vi "Reliability Project MAIN (PC).vi"() -> ()   [LabVIEW 2019]
uses:
  TypeDef/Test Header.ctl
  TypeDef/Graph Parameters.ctl
  TypeDef/Color.ctl
  TypeDef/Graph Type.ctl
  TypeDef/Graph Output File.ctl
  TypeDef/Test Style.ctl
  TCP/PC/Event Mode.ctl
  TypeDef/Config.ctl
  TypeDef/Test Config.ctl
  TypeDef/Test Parameters.ctl
  <vilib>/Utility/miscctls.llb/LVDateTimeRec.ctl
  TCP/PC/PCsend RTrecv CMD.ctl
  TypeDef/ConnSettingCluster.ctl
  <vilib>/Utility/file.llb/Read Delimited Spreadsheet (DBL).vi
  <vilib>/Utility/config.llb/NI_LVConfig.lvlib
  <vilib>/Utility/config.llb/Write Key (Boolean).vi
  <resource>/objmgr/ni.dex.rc
panel:
  in  "Screen":T1(tab)
  in  "Run Test Tab":enum32{"Page 1"}(tab)
  out "Chart":dbl[][](graph)=[[-0.00241851806640625, 9.5367431640625e-05, 2.3512725830078125, 5.211483001708984, 5.211483001708984], [-0.0020904541015625, 0.0007476806640625, 2.350067138671875, 5.209384918212891, 5.209384918212891], [-0.00305938720703125, 0.00110626220703125, 2.350513458251953, 5.209739685058594, 5.209739685058594], [-0.0022525787353515625, 0.000324249267578125, 2.350391387939453, 5.2073822021484375, 5.2073822021484375], [-0.002140045166015625, 0.0006237030029296875, 2.3496646881103516, 5.206989288330078, 5.206989288330078], [-0.00235748291015625, 0.0009613037109375, 2.349153518676758, 5.206110000610352, 5.206110000610352], [-0.0056972503662109375, -0.000194549560546875, 2.3493595123291016, 5.206518173217773, 5.206518173217773], [-0.002033233642578125, 0.0008106231689453125, 2.347330093383789, 5.203701019287109, 5.203701019287109], [-0.00220489501953125, 0.0001850128173828125, 2.3487815856933594, 5.203361511230469, 5.203361511230469], [-0.002315521240234375, 0.0008544921875, 2.348348617553711, 5.2019500732421875, 5.2019500732421875], [-0.0024318695068359375, 0.0006542205810546875, 2.3473949432373047, 5.201688766479492, 5.201688766479492], [-0.0023937225341796875, 0.0006656646728515625, 2.3465042114257812, 5.199775695800781, 5.199775695800781], [-0.002849578857421875, 0.001049041748046875, 2.346738815307617, 5.199516296386719, 5.199516296386719], [-0.0024662017822265625, 0.001140594482421875, 2.3461246490478516, 5.19781494140625, 5.19781494140625], [-0.0017299652099609375, -0.0011444091796875, 2.3457717895507812, 5.19737434387207, 5.19737434387207], [-0.0023097991943359375, 0.0001659393310546875, 2.345857620239258, 5.196210861206055, 5.196210861206055], [-0.0028095245361328125, 0.0006008148193359375, 2.3449745178222656, 5.195291519165039, 5.195291519165039], [-0.0024776458740234375, 0.0011157989501953125, 2.342325210571289, 5.194158554077148, 5.194158554077148], [-0.0025463104248046875, 0.0005931854248046875, 2.344541549682617, 5.193063735961914, 5.193063735961914], [0.00582122802734375, 8.392333984375e-05, 2.3436336517333984, 5.192634582519531, 5.192634582519531], [-0.004276275634765625, 0.0004634857177734375, 2.3434505462646484, 5.190740585327148, 5.190740585327148], [-0.00257110595703125, 0.0012760162353515625, 2.342508316040039, 5.190359115600586, 5.190359115600586], [-0.0032100677490234375, 0.0006885528564453125, 2.3427352905273438, 5.188653945922852, 5.188653945922852], [-0.0021190643310546875, 0.0008945465087890625, 2.3419570922851562, 5.188499450683594, 5.188499450683594], [-0.0022907257080078125, 0.000335693359375, 2.3421077728271484, 5.186103820800781, 5.186103820800781], [-0.0024394989013671875, 0.0010929107666015625, 2.3413314819335938, 5.186931610107422, 5.186931610107422], [-0.00225830078125, 0.0002803802490234375, 2.3414478302001953, 5.183507919311523, 5.183507919311523], [-0.0024089813232421875, 0.0014781951904296875, 2.340656280517578, 5.184579849243164, 5.184579849243164], [-0.002437591552734375, 0.0005931854248046875, 2.3399314880371094, 5.182092666625977, 5.182092666625977], [-0.002262115478515625, 0.0003643035888671875, 2.3407840728759766, 5.182659149169922, 5.182659149169922], [-0.0025005340576171875, -0.000225067138671875, 2.3396263122558594, 5.1800079345703125, 5.1800079345703125], [-0.00218963623046875, 0.0027942657470703125, 2.338764190673828, 5.180774688720703, 5.180774688720703], [-0.0020732879638671875, 0.0009441375732421875, 2.3374996185302734, 5.177848815917969, 5.177848815917969], [-0.001556396484375, 0.0001373291015625, 2.338285446166992, 5.178548812866211, 5.178548812866211], [-0.0018310546875, 0.0006046295166015625, 2.3379344940185547, 5.175708770751953, 5.175708770751953], [-0.0020771026611328125, 0.0011043548583984375, 2.337373733520508, 5.1764984130859375, 5.1764984130859375], [-0.0024662017822265625, 0.0002307891845703125, 2.3374977111816406, 5.174013137817383, 5.174013137817383], [-0.0022106170654296875, 0.0005321502685546875, 2.336719512939453, 5.174356460571289, 5.174356460571289], [-0.002288818359375, 0.00014495849609375, 2.3338546752929688, 5.171659469604492, 5.171659469604492], [-0.00229644775390625, 0.00081634521484375, 2.335407257080078, 5.172262191772461, 5.172262191772461], [-0.002166748046875, 0.0012416839599609375, 2.327573776245117, 5.169179916381836, 5.169179916381836], [-0.002197265625, 0.000247955322265625, 2.3348464965820312, 5.169887542724609, 5.169887542724609], [-0.002292633056640625, 0.0009975433349609375, 2.334583282470703, 5.167793273925781, 5.167793273925781], [-0.002685546875, 0.0006885528564453125, 2.333953857421875, 5.167308807373047, 5.167308807373047], [-0.002529144287109375, 0.00035858154296875, 2.3336315155029297, 5.165552139282227, 5.165552139282227], [-0.0021762847900390625, 0.0009937286376953125, 2.33294677734375, 5.165216445922852, 5.165216445922852], [-0.002208709716796875, 0.00069427490234375, 2.33135986328125, 5.163597106933594, 5.163597106933594], [-0.0024356842041015625, 0.0005512237548828125, 2.3313236236572266, 5.163679122924805, 5.163679122924805], [-0.002361297607421875, -0.000225067138671875, 2.3319091796875, 5.161943435668945, 5.161943435668945], [-0.0022907257080078125, -0.002529144287109375, 2.3310108184814453, 5.161035537719727, 5.161035537719727], [-0.00202178955078125, 0.0004749298095703125, 2.331541061401367, 5.15962028503418, 5.15962028503418], [-0.00238037109375, -3.0517578125e-05, 2.330432891845703, 5.1588134765625, 5.1588134765625], [-0.001461029052734375, 0.000629425048828125, 2.3308582305908203, 5.157678604125977, 5.157678604125977], [-0.0025424957275390625, 0.0003337860107421875, 2.329559326171875, 5.156576156616211, 5.156576156616211], [-0.002460479736328125, 0.00069427490234375, 2.3291893005371094, 5.156003952026367, 5.156003952026367], [-0.0024356842041015625, 0.001369476318359375, 2.328702926635742, 5.154455184936523, 5.154455184936523], [-0.00209808349609375, 0.00127410888671875, 2.328824996948242, 5.154962539672852, 5.154962539672852], [-0.001079559326171875, 0.0003757476806640625, 2.329326629638672, 5.152063369750977, 5.152063369750977], [-0.0030384063720703125, 0.0001125335693359375, 2.3291149139404297, 5.152074813842773, 5.152074813842773], [-0.0016727447509765625, 5.91278076171875e-05, 2.329296112060547, 5.149860382080078, 5.149860382080078], [-0.002384185791015625, 0.0006103515625, 2.3267383575439453, 5.150243759155273, 5.150243759155273], [-0.00270843505859375, -9.5367431640625e-05, 2.325765609741211, 5.147882461547852, 5.147882461547852], [-0.0021114349365234375, 0.0008640289306640625, 2.325572967529297, 5.148151397705078, 5.148151397705078], [-0.00231170654296875, 0.0012378692626953125, 2.325998306274414, 5.145776748657227, 5.145776748657227], [-0.001338958740234375, 0.0006275177001953125, 2.325258255004883, 5.146303176879883, 5.146303176879883], [-0.0024394989013671875, 0.0006237030029296875, 2.3251724243164062, 5.143526077270508, 5.143526077270508], [-0.0023479461669921875, 0.0012683868408203125, 2.323986053466797, 5.143976211547852, 5.143976211547852], [-0.002422332763671875, 0.0004558563232421875, 2.3242645263671875, 5.1414794921875, 5.1414794921875], [0.0050868988037109375, 0.0001163482666015625, 2.3232860565185547, 5.141656875610352, 5.141656875610352], [-0.0023784637451171875, -2.86102294921875e-05, 2.323179244995117, 5.140108108520508, 5.140108108520508], [-0.0021877288818359375, 0.0002689361572265625, 2.322599411010742, 5.139678955078125, 5.139678955078125], [-0.0022735595703125, 0.000621795654296875, 2.3229293823242188, 5.137945175170898, 5.137945175170898], [-0.002384185791015625, 0.0003204345703125, 2.3215789794921875, 5.137645721435547, 5.137645721435547], [-0.002407073974609375, 0.0003681182861328125, 2.3217506408691406, 5.1365814208984375, 5.1365814208984375], [-0.0019683837890625, 0.000946044921875, 2.3209781646728516, 5.136013031005859, 5.136013031005859], [-0.002208709716796875, 0.000820159912109375, 2.320514678955078, 5.134279251098633, 5.134279251098633], [-0.002262115478515625, 0.0007038116455078125, 2.320322036743164, 5.133800506591797, 5.133800506591797], [-0.0022068023681640625, 0.000804901123046875, 2.3203296661376953, 5.132570266723633, 5.132570266723633], [-0.0026531219482421875, 0.000782012939453125, 2.318910598754883, 5.131275177001953, 5.131275177001953], [-0.0024929046630859375, 0.00089263916015625, 2.3195762634277344, 5.130367279052734, 5.130367279052734], [-0.00217437744140625, 0.000827789306640625, 2.3187484741210938, 5.129323959350586, 5.129323959350586], [-0.0023651123046875, 0.0007495880126953125, 2.3187007904052734, 5.128835678100586, 5.128835678100586], [-0.0020999908447265625, 0.00095367431640625, 2.3181400299072266, 5.127468109130859, 5.127468109130859], [-0.0024890899658203125, 0.0009746551513671875, 2.3181591033935547, 5.12727165222168, 5.12727165222168], [-0.0021305084228515625, 0.00098419189453125, 2.3174896240234375, 5.125310897827148, 5.125310897827148], [-0.002712249755859375, 0.0005664825439453125, 2.3167991638183594, 5.125190734863281, 5.125190734863281], [-0.0021343231201171875, 0.0006313323974609375, 2.3164443969726562, 5.123414993286133, 5.123414993286133], [-0.0029354095458984375, 0.0004596710205078125, 2.3162708282470703, 5.123697280883789, 5.123697280883789], [-0.00228118896484375, -7.62939453125e-06, 2.3158607482910156, 5.121555328369141, 5.121555328369141], [-0.0022182464599609375, 0.0007076263427734375, 2.3154754638671875, 5.12164306640625, 5.12164306640625], [-0.002349853515625, 0.0007724761962890625, 2.315549850463867, 5.119346618652344, 5.119346618652344], [-0.002269744873046875, 0.001094818115234375, 2.3123722076416016, 5.119991302490234, 5.119991302490234], [-0.00231170654296875, 0.0002613067626953125, 2.3144569396972656, 5.117624282836914, 5.117624282836914], [-0.00157928466796875, 0.000156402587890625, 2.313823699951172, 5.118106842041016, 5.118106842041016], [-0.0027179718017578125, 0.0005702972412109375, 2.314136505126953, 5.115741729736328, 5.115741729736328], [-0.0025234222412109375, 3.814697265625e-06, 2.312936782836914, 5.116338729858398, 5.116338729858398], [-0.002349853515625, 0.0016937255859375, 2.3126564025878906, 5.113800048828125, 5.113800048828125], [-0.0027751922607421875, 0.0006504058837890625, 2.312501907348633, 5.1144256591796875, 5.1144256591796875], [-0.002429962158203125, 0.00086212158203125, 2.31304931640625, 5.112766265869141, 5.112766265869141], [-0.0024261474609375, 0.0006504058837890625, 2.3119125366210938, 5.112785339355469, 5.112785339355469], [-0.0024738311767578125, -1.33514404296875e-05, 2.3113555908203125, 5.110126495361328, 5.110126495361328], [-0.002063751220703125, 4.76837158203125e-05, 2.308307647705078, 5.110754013061523, 5.110754013061523], [-0.00232696533203125, -6.103515625e-05, 2.31024169921875, 5.108325958251953, 5.108325958251953], [-0.002197265625, 0.00018310546875, 2.3096885681152344, 5.109380722045898, 5.109380722045898], [-0.0021686553955078125, 0.000545501708984375, 2.3098373413085938, 5.106624603271484, 5.106624603271484], [-0.0011692047119140625, 0.000392913818359375, 2.309000015258789, 5.107295989990234, 5.107295989990234], [-0.0025653839111328125, 0.0001506805419921875, 2.3094406127929688, 5.105155944824219, 5.105155944824219], [-0.002166748046875, 0.000545501708984375, 2.3088741302490234, 5.105400085449219, 5.105400085449219], [-0.00229644775390625, 0.000518798828125, 2.3076095581054688, 5.102983474731445, 5.102983474731445], [-0.0026874542236328125, 0.00115966796875, 2.3078269958496094, 5.103851318359375, 5.103851318359375], [-0.0022907257080078125, 0.0001049041748046875, 2.308218002319336, 5.101722717285156, 5.101722717285156], [-0.0018825531005859375, 0.000579833984375, 2.3090286254882812, 5.102010726928711, 5.102010726928711], [-0.002620697021484375, 0.000263214111328125, 2.3078346252441406, 5.100181579589844, 5.100181579589844], [-0.0020904541015625, 0.000461578369140625, 2.3070220947265625, 5.09980583190918, 5.09980583190918], [-0.002315521240234375, 8.96453857421875e-05, 2.2959556579589844, 5.099071502685547, 5.099071502685547], [-0.0024433135986328125, -3.4332275390625e-05, 2.306089401245117, 5.098339080810547, 5.098339080810547], [-0.0015163421630859375, 1.52587890625e-05, 2.305643081665039, 5.097761154174805, 5.097761154174805], [-0.00197601318359375, 0.0005550384521484375, 2.305318832397461, 5.096200942993164, 5.096200942993164], [-0.002300262451171875, 0.0008144378662109375, 2.3057098388671875, 5.096399307250977, 5.096399307250977], [-0.0022907257080078125, 0.001064300537109375, 2.304637908935547, 5.094629287719727, 5.094629287719727], [-0.0023441314697265625, 0.000896453857421875, 2.3045883178710938, 5.094669342041016, 5.094669342041016], [-0.0025272369384765625, 0.0006122589111328125, 2.3042259216308594, 5.092912673950195, 5.092912673950195], [-0.002017974853515625, 0.000339508056640625, 2.303884506225586, 5.093050003051758, 5.093050003051758], [-0.0024871826171875, 0.000335693359375, 2.3036632537841797, 5.091398239135742, 5.091398239135742], [-0.0026378631591796875, 0.0004863739013671875, 2.291349411010742, 5.092126846313477, 5.092126846313477], [-0.0020580291748046875, 0.0008220672607421875, 2.303516387939453, 5.089519500732422, 5.089519500732422], [-0.0019683837890625, 0.0003223419189453125, 2.302806854248047, 5.090400695800781, 5.090400695800781], [-0.00337982177734375, 0.0012302398681640625, 2.3025283813476562, 5.087850570678711, 5.087850570678711], [-0.0022869110107421875, 0.0002040863037109375, 2.299816131591797, 5.088750839233398, 5.088750839233398], [-0.0024471282958984375, 0.0006580352783203125, 2.302255630493164, 5.086374282836914, 5.086374282836914], [-0.0022602081298828125, 0.0002288818359375, 2.301565170288086, 5.087335586547852, 5.087335586547852], [-0.002094268798828125, -3.4332275390625e-05, 2.300901412963867, 5.085031509399414, 5.085031509399414], [-0.0021820068359375, 0.0004425048828125, 2.300508499145508, 5.085823059082031, 5.085823059082031], [-0.003513336181640625, -0.00026702880859375, 2.3003177642822266, 5.0836639404296875, 5.0836639404296875], [-0.0021228790283203125, 0.00023651123046875, 2.299711227416992, 5.084384918212891, 5.084384918212891], [-0.0023136138916015625, 7.62939453125e-05, 2.3003311157226562, 5.082035064697266, 5.082035064697266], [-0.002285003662109375, 2.288818359375e-05, 2.2995033264160156, 5.083127975463867, 5.083127975463867], [-0.0023632049560546875, 0.00054931640625, 2.2997283935546875, 5.080684661865234, 5.080684661865234], [-0.0022487640380859375, 0.000881195068359375, 2.299091339111328, 5.081302642822266, 5.081302642822266], [-0.00244903564453125, 0.0009021759033203125, 2.2994842529296875, 5.079761505126953, 5.079761505126953], [-0.00209808349609375, 0.000762939453125, 2.2970943450927734, 5.080654144287109, 5.080654144287109], [-0.0023212432861328125, 4.38690185546875e-05, 2.3003578186035156, 5.078205108642578, 5.078205108642578], [-0.0018157958984375, 0.0008544921875, 2.2980213165283203, 5.078620910644531, 5.078620910644531], [-0.0022640228271484375, 0.0011501312255859375, 2.2982006072998047, 5.0772857666015625, 5.0772857666015625], [-0.0029888153076171875, 0.0002002716064453125, 2.298887252807617, 5.07684326171875, 5.07684326171875], [-0.0024242401123046875, 0.0006103515625, 2.2978076934814453, 5.075416564941406, 5.075416564941406], [-0.0022754669189453125, 0.0011653900146484375, 2.297220230102539, 5.0757904052734375, 5.0757904052734375], [-0.001163482666015625, 0.0010986328125, 2.297616958618164, 5.07489013671875, 5.07489013671875], [-0.002658843994140625, 0.0008525848388671875, 2.2969589233398438, 5.074573516845703, 5.074573516845703], [-0.0022487640380859375, 0.0010128021240234375, 2.2956104278564453, 5.073554992675781, 5.073554992675781], [-0.0024967193603515625, 0.0009746551513671875, 2.296297073364258, 5.073375701904297, 5.073375701904297], [-0.0025348663330078125, -0.0001773834228515625, 2.2911739349365234, 5.07227897644043, 5.07227897644043], [-0.0026683807373046875, 0.00122833251953125, 2.297945022583008, 5.072353363037109, 5.072353363037109], [-0.0019474029541015625, 0.0010662078857421875, 2.2958545684814453, 5.071252822875977, 5.071252822875977], [-0.002422332763671875, 0.000732421875, 2.295177459716797, 5.071023941040039, 5.071023941040039], [-0.00240325927734375, -0.0006256103515625, 2.295278549194336, 5.070167541503906, 5.070167541503906], [-0.00270843505859375, 0.0004940032958984375, 2.2949085235595703, 5.070009231567383, 5.070009231567383], [-0.0024509429931640625, 0.0009822845458984375, 2.295053482055664, 5.06922721862793, 5.06922721862793], [-0.0033931732177734375, 3.4332275390625e-05, 2.294820785522461, 5.068716049194336, 5.068716049194336], [-0.0019702911376953125, 0.0010128021240234375, 2.2952404022216797, 5.068096160888672, 5.068096160888672], [-0.0023193359375, 0.0004405975341796875, 2.294109344482422, 5.067258834838867, 5.067258834838867], [-0.0024013519287109375, 0.00025177001953125, 2.2938690185546875, 5.067533493041992, 5.067533493041992], [-0.00215911865234375, 0.00032806396484375, 2.2927303314208984, 5.066440582275391, 5.066440582275391], [-0.001934051513671875, 0.000698089599609375, 2.2940006256103516, 5.066160202026367, 5.066160202026367], [-0.00247955322265625, 0.0002422332763671875, 2.293081283569336, 5.065158843994141, 5.065158843994141], [-0.00244903564453125, 0.0005702972412109375, 2.292530059814453, 5.065837860107422, 5.065837860107422], [-0.002269744873046875, 0.00032806396484375, 2.2919998168945312, 5.064092636108398, 5.064092636108398], [-0.0024890899658203125, 0.0002803802490234375, 2.292816162109375, 5.064476013183594, 5.064476013183594], [-0.0021076202392578125, 0.0007839202880859375, 2.2923927307128906, 5.063138961791992, 5.063138961791992], [-0.0026073455810546875, 0.0004119873046875, 2.292522430419922, 5.0640716552734375, 5.0640716552734375], [-0.0022125244140625, 0.0003604888916015625, 2.292064666748047, 5.061803817749023, 5.061803817749023], [-0.0021190643310546875, 0.00043487548828125, 2.291830062866211, 5.063020706176758, 5.063020706176758], [-0.0026988983154296875, -8.58306884765625e-05, 2.291942596435547, 5.060863494873047, 5.060863494873047], [-0.0024967193603515625, 0.0013103485107421875, 2.2912254333496094, 5.062192916870117, 5.062192916870117], [-0.0023708343505859375, 0.0013580322265625, 2.290983200073242, 5.060268402099609, 5.060268402099609], [-0.0019283294677734375, 0.0005130767822265625, 2.2912445068359375, 5.0613250732421875, 5.0613250732421875], [-0.00235748291015625, 0.0006389617919921875, 2.291158676147461, 5.059490203857422, 5.059490203857422], [-0.0021953582763671875, 0.0008640289306640625, 2.290618896484375, 5.060487747192383, 5.060487747192383], [-0.002262115478515625, 0.0003376007080078125, 2.2910594940185547, 5.058900833129883, 5.058900833129883], [-0.004283905029296875, 0.0003986358642578125, 2.2887744903564453, 5.059345245361328, 5.059345245361328], [-0.0024280548095703125, 0.00084686279296875, 2.2905349731445312, 5.057645797729492, 5.057645797729492], [-0.0024051666259765625, 0.001026153564453125, 2.289949417114258, 5.0586395263671875, 5.0586395263671875], [-0.00244140625, 0.0017452239990234375, 2.2903308868408203, 5.056642532348633, 5.056642532348633], [-0.0020580291748046875, 0.0011138916015625, 2.2884883880615234, 5.057493209838867, 5.057493209838867], [-0.00202178955078125, 0.0007648468017578125, 2.2892799377441406, 5.055974960327148, 5.055974960327148], [-0.0024394989013671875, -8.7738037109375e-05, 2.289255142211914, 5.057348251342773, 5.057348251342773], [-0.0016193389892578125, 0.0003337860107421875, 2.288480758666992, 5.055501937866211, 5.055501937866211], [-0.0021190643310546875, 0.000507354736328125, 2.2884178161621094, 5.056310653686523, 5.056310653686523], [-0.002429962158203125, 0.001087188720703125, 2.2895164489746094, 5.05482292175293, 5.05482292175293], [-0.002117156982421875, 0.000701904296875, 2.2885704040527344, 5.055061340332031, 5.055061340332031], [-0.0021724700927734375, 0.000560760498046875, 2.2890186309814453, 5.054107666015625, 5.054107666015625], [-0.002399444580078125, 0.00107574462890625, 2.2880687713623047, 5.054941177368164, 5.054941177368164], [-0.00286865234375, 0.000347137451171875, 2.288494110107422, 5.053903579711914, 5.053903579711914], [-0.0020732879638671875, 0.000972747802734375, 2.288127899169922, 5.053012847900391, 5.053012847900391], [-0.00222015380859375, 0.0010051727294921875, 2.2885360717773438, 5.053804397583008, 5.053804397583008], [-0.002368927001953125, 0.0002231597900390625, 2.288074493408203, 5.053201675415039, 5.053201675415039], [-0.0024871826171875, 0.0008525848388671875, 2.28802490234375, 5.0528564453125, 5.0528564453125], [-0.00225067138671875, 0.0009307861328125, 2.2883853912353516, 5.052770614624023, 5.052770614624023], [-0.0021457672119140625, 0.0007495880126953125, 2.287994384765625, 5.051923751831055, 5.051923751831055], [-0.0021305084228515625, 0.0013179779052734375, 2.28741455078125, 5.051168441772461, 5.051168441772461]]
  in  "pb.graph control":bool caption="Digital Output 4"
  in  "pb.RunSweeps":bool caption="Start Sweeps"
  out "Abs. Height":dbl
  out "PS Volt":dbl
  out "LS Volt":dbl
  out "Spare":dbl
  in  "Sweep Time (s)":dbl min=0.0 step=0.01 format="%.2g"
  in  "Sweep End Height":dbl
  in  "Number of Sweeps":i32
  out "Data Path":path
  in  "Sweep Start Height":dbl
  in  "Sweep PS Cmd":dbl
  out "Resistance":dbl=nan
  out "Sweeps Complete":i16
  out "Min Height":dbl
  out "Max Height":dbl
  in  "Spare Output":dbl
  in  "PS Command":dbl
  in  "Position Command":dbl=nan
  in  "pb.TareHeight":bool caption="Start Sweeps"
  out "Relative Height":dbl format="%#.3g"
  in  "Test Setup Tab":enum32{"Page 1"}(tab)
  in  "pb.Open Test Config":bool caption="Copy Test Setup"
  out "Test Config":string
  in  "Test Style":T2
  in  "Bias Resistance":dbl=nan
  in  "pb.Copy Test Config":bool caption="Copy Test Setup"
  in  "Graph Setup Tab":enum32{"Page 1"}(tab)
  in  "pb.Graph by File":bool caption="Digital Output 4"
  in  "pb.Re-Run Graph":bool caption="Digital Output 4"
  in  "Graph Parameters":T3={"Tol Path"=path "", "Tol Band Color"=enum."Red", "Graph Type"=enum."H vs R (1 Cycle)", "Height Min"=0, "Height Max"=0, "Height Interval"=0, "Res Max"=0, "Res Interval"=0, "Time Max"=0, "Time Interval"=0, "Graph Output File"=enum."pdf", "Auto Open"=TRUE}
  in  "Test Header Tab":enum32{"Page 1"}(tab)
  in  "Test Header":T7
  out "led.DataWarning":bool=TRUE caption="Check last file for missing data\n          (jumps in height)"
  in  "pb.CalPage":bool caption="Digital Output 4"
  out "IP Address":string
  in  "pb.connect":bool
  out "InvalidResponses":string
  out "Error Out":errorcluster
  in  "FlattenedData":string
  in  "Command":string
  in  "Connected?":bool
  in  "Connected? 2":bool
  in  "Panel Close?":bool
  in  "pb.DO0":bool caption="Digital Output 1"
  in  "pb.DO1":bool caption="Digital Output 2"
  in  "pb.DO2":bool caption="Digital Output 3"
  in  "pb.DO3":bool caption="Digital Output 4"
  out "led.DI 4":bool caption="Digital Input 1"
  out "led.DI 5":bool caption="Digital Input 2"
  out "led.DI 6":bool caption="Digital Input 3"
  out "led.DI 7":bool caption="Digital Input 4"
  in  "Cal Due Date:":timestamp=timestamp(3029616000 s since 1904-01-01) format="%<%m/%d/%y>T"
  in  "Gauge Number:":i32[](array[numeric])=[0, 0, 0, 0, 0, 0, 0]
  out "Cal Readings:":dbl[](array[numeric])
  in  "Cal Controls:":dbl[](array[numeric])=[nan, 0.0, 0.0]
  in  "pb.RevertCal":bool
  in  "pb.SaveCal":bool
  out "Channels:":string[](array[string])=["Power Supply Voltage", "Level Sender Voltage", "AI-3 Spare", "Height Gauge", "Position Command", "Power Supply Command", "Spare Output"]
  in  "Offset Values:":dbl[](array[numeric])=[0.0, 0.0, 0.0, 0.0, 0.0, 0.0, 0.0]
  in  "Slope Values:":dbl[](array[numeric])=[0.0, 0.0, 0.0, 0.0, 0.0, 0.0, 0.0]
  in  "pb.RunScreen":bool caption="Digital Output 4"
  # "Run Test"
  # "Test Setup"
  # "Graph Setup"
  # "Test Header"
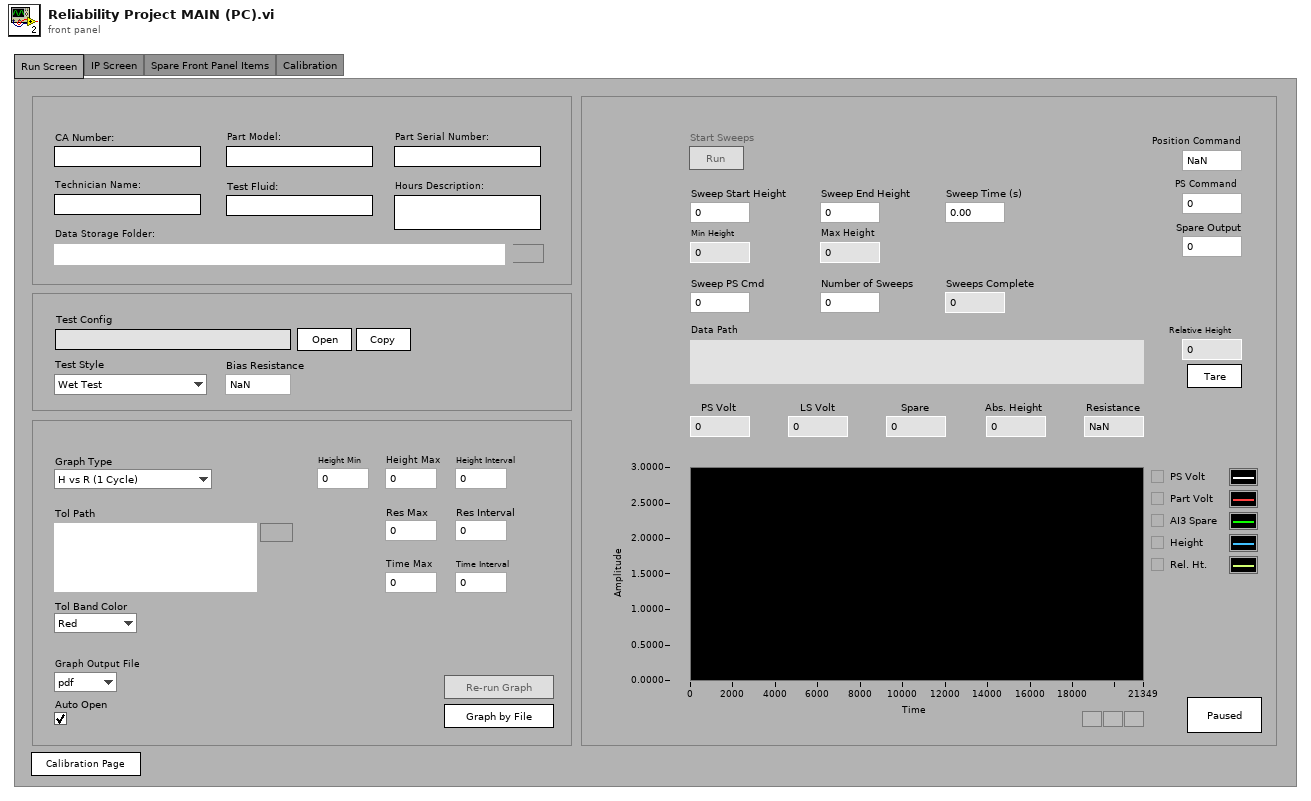
[diagram p1: front panel]
types:
  T1 = enum32{"Run Screen", "IP Screen", "Spare Front Panel Items", "Calibration"}
  T2 = typedef "Test Style.ctl" = enum16{"Wet Test", "Dry Test", "Contact Test"}
  T3 = typedef "Graph Parameters.ctl" = cluster{"Tol Path":path, "Tol Band Color":T4, "Graph Type":T5, "Height Min":i32, "Height Max":i32, "Height Interval":i32, "Res Max":i32, "Res Interval":i32, "Time Max":i32, "Time Interval":i32, "Graph Output File":T6, "Auto Open":bool}
  T4 = typedef "Color.ctl" = enum16{"Red", "Black", "Green", "Blue", "Orange", "Yellow", "Purple", "Grey"}
  T5 = typedef "Graph Type.ctl" = enum16{"H vs R (1 Cycle)", "T vs R (Multiple Cycles)", "H vs R & T vs R (1 Cycle)"}
  T6 = typedef "Graph Output File.ctl" = enum16{"png", "pdf"}
  T7 = typedef "Test Header.ctl" = cluster{"CA Number:":string, "Part Model:":string, "Part Serial Number:":string, "Technician Name:":string, "Test Fluid:":string, "Hours Description:":string, "Data Storage Folder:":path}
  T8 = typedef "Test Config.ctl" = cluster{"Test Header":T7, "Test Style":T2, "Bias Resistance":dbl, "Height Offset":dbl, "Graph Parameters":T3, "Test Parameters":T9}
  T9 = typedef "Test Parameters.ctl" = cluster{"Sweep Start Height":dbl, "Sweep End Height":dbl, "Sweep Time (s)":dbl, "Sweep PS Cmd":dbl, "Number of Sweeps":i32}
  T10 = typedef "Config.ctl" = cluster{"Test Config Path":path, "RT IP Address":string}
  T11 = typedef "Event Mode.ctl" = enum16{"Init", "Get", "Set", "Destroy"}
  T12 = cluster{"Config":T10, "RIOTries":i32, "RIOconnection":bool, "IP Address":string, "ValidFile?":bool, "Graph Active":bool, "Data Clock":dbl, "Data Timing":dbl, "Data":dbl[][], "Data_Current":dbl[], "Slope Values":dbl[], "Offset Values":dbl[], "Controls":dbl[], "Height Offset":dbl, "Data Path":path, "SweepsRunning":bool, "SweepsForward":bool, "SweepsSwept":i32, "Gauge#":i32, "CalDueDate":string, "Data Index":i32, "Sweep Clock":dbl, "Sweep Timing":dbl, "Waveform":dbl[], "Wave.pts":i32, "Current Point":i32, "FinalizeSweeps":bool, "New Data":bool, "MaxResistance":dbl, "Min Height":dbl, "Max Height":dbl, "Graph Time":dbl, "Config Path":path, "Time v Res":bool, "Test Params":T8, "Test Config":string, "Graphing Script Dir":path, "Graph Data":dbl[][]}
  T13 = typedef "LVDateTimeRec.ctl" = cluster{"fractional second":dbl, "second":i32, "minute":i32, "hour":i32, "day of month":i32, "month":i32, "year":i32, "day of week":i32, "day of year":i32, "DST":i32}
  T14 = typedef "PCsend RTrecv CMD.ctl" = enum16{"ConnSettings", "Connect", "Stop", "Digital Outputs", "Analog Outputs", "Sweep Parameters", "Start Sweep", "Cal2RT", "Save Cal", "Load Cal"}
  T15 = enum32{"Run Screen", "IP Screen", "Spare Front Panel Items", "Calibration", "New LS"}
  T16 = enum32{"invalid app kind", "Development System", "Run Time System", "Student Edition", "Embedded LabVIEW", "Evaluation", "Custom"}
  T17 = enum16{"Read Data", "Write Data", "Write Cal", "Init", "Write Stream Error"}
  T18 = cluster{"Slope":dbl[], "Offset":dbl[], "Gauge#":i32, "CalDueDate":string}
  T19 = enum16{"open", "replace", "create", "open or create", "replace or create", "replace or create with confirmation"}
  T20 = enum8{"Enabled", "Disabled", "Disabled and Grayed Out"}
  T21 = enum32{"Run Screen", "Test Configuration Page", "Stand Configuration Page", "RIO Connection", "Part Change", "Spare Front Panel Items", "Intro", "Cal Warning"}
  T22 = typedef "RTsend PCrecv CMD.ctl" = enum16{"Digital Inputs", "Connected?", "Data", "Data 2", "Cal2PC"}
  T23 = cluster{"Slope Values":dbl[], "Offset Values":dbl[]}
  T24 = cluster{"Numeric":i32, "date/time string":string}
  T25 = typedef "NI_LVConfig.lvlib/Config Data RefNum.ctl" = refnum<k1>
  T26 = typedef "ConnSettingCluster.ctl" = cluster{"ConnectAttemptLimit(5)":u32, "IP Address":string, "Send Port":u16, "Recv Port":u16}
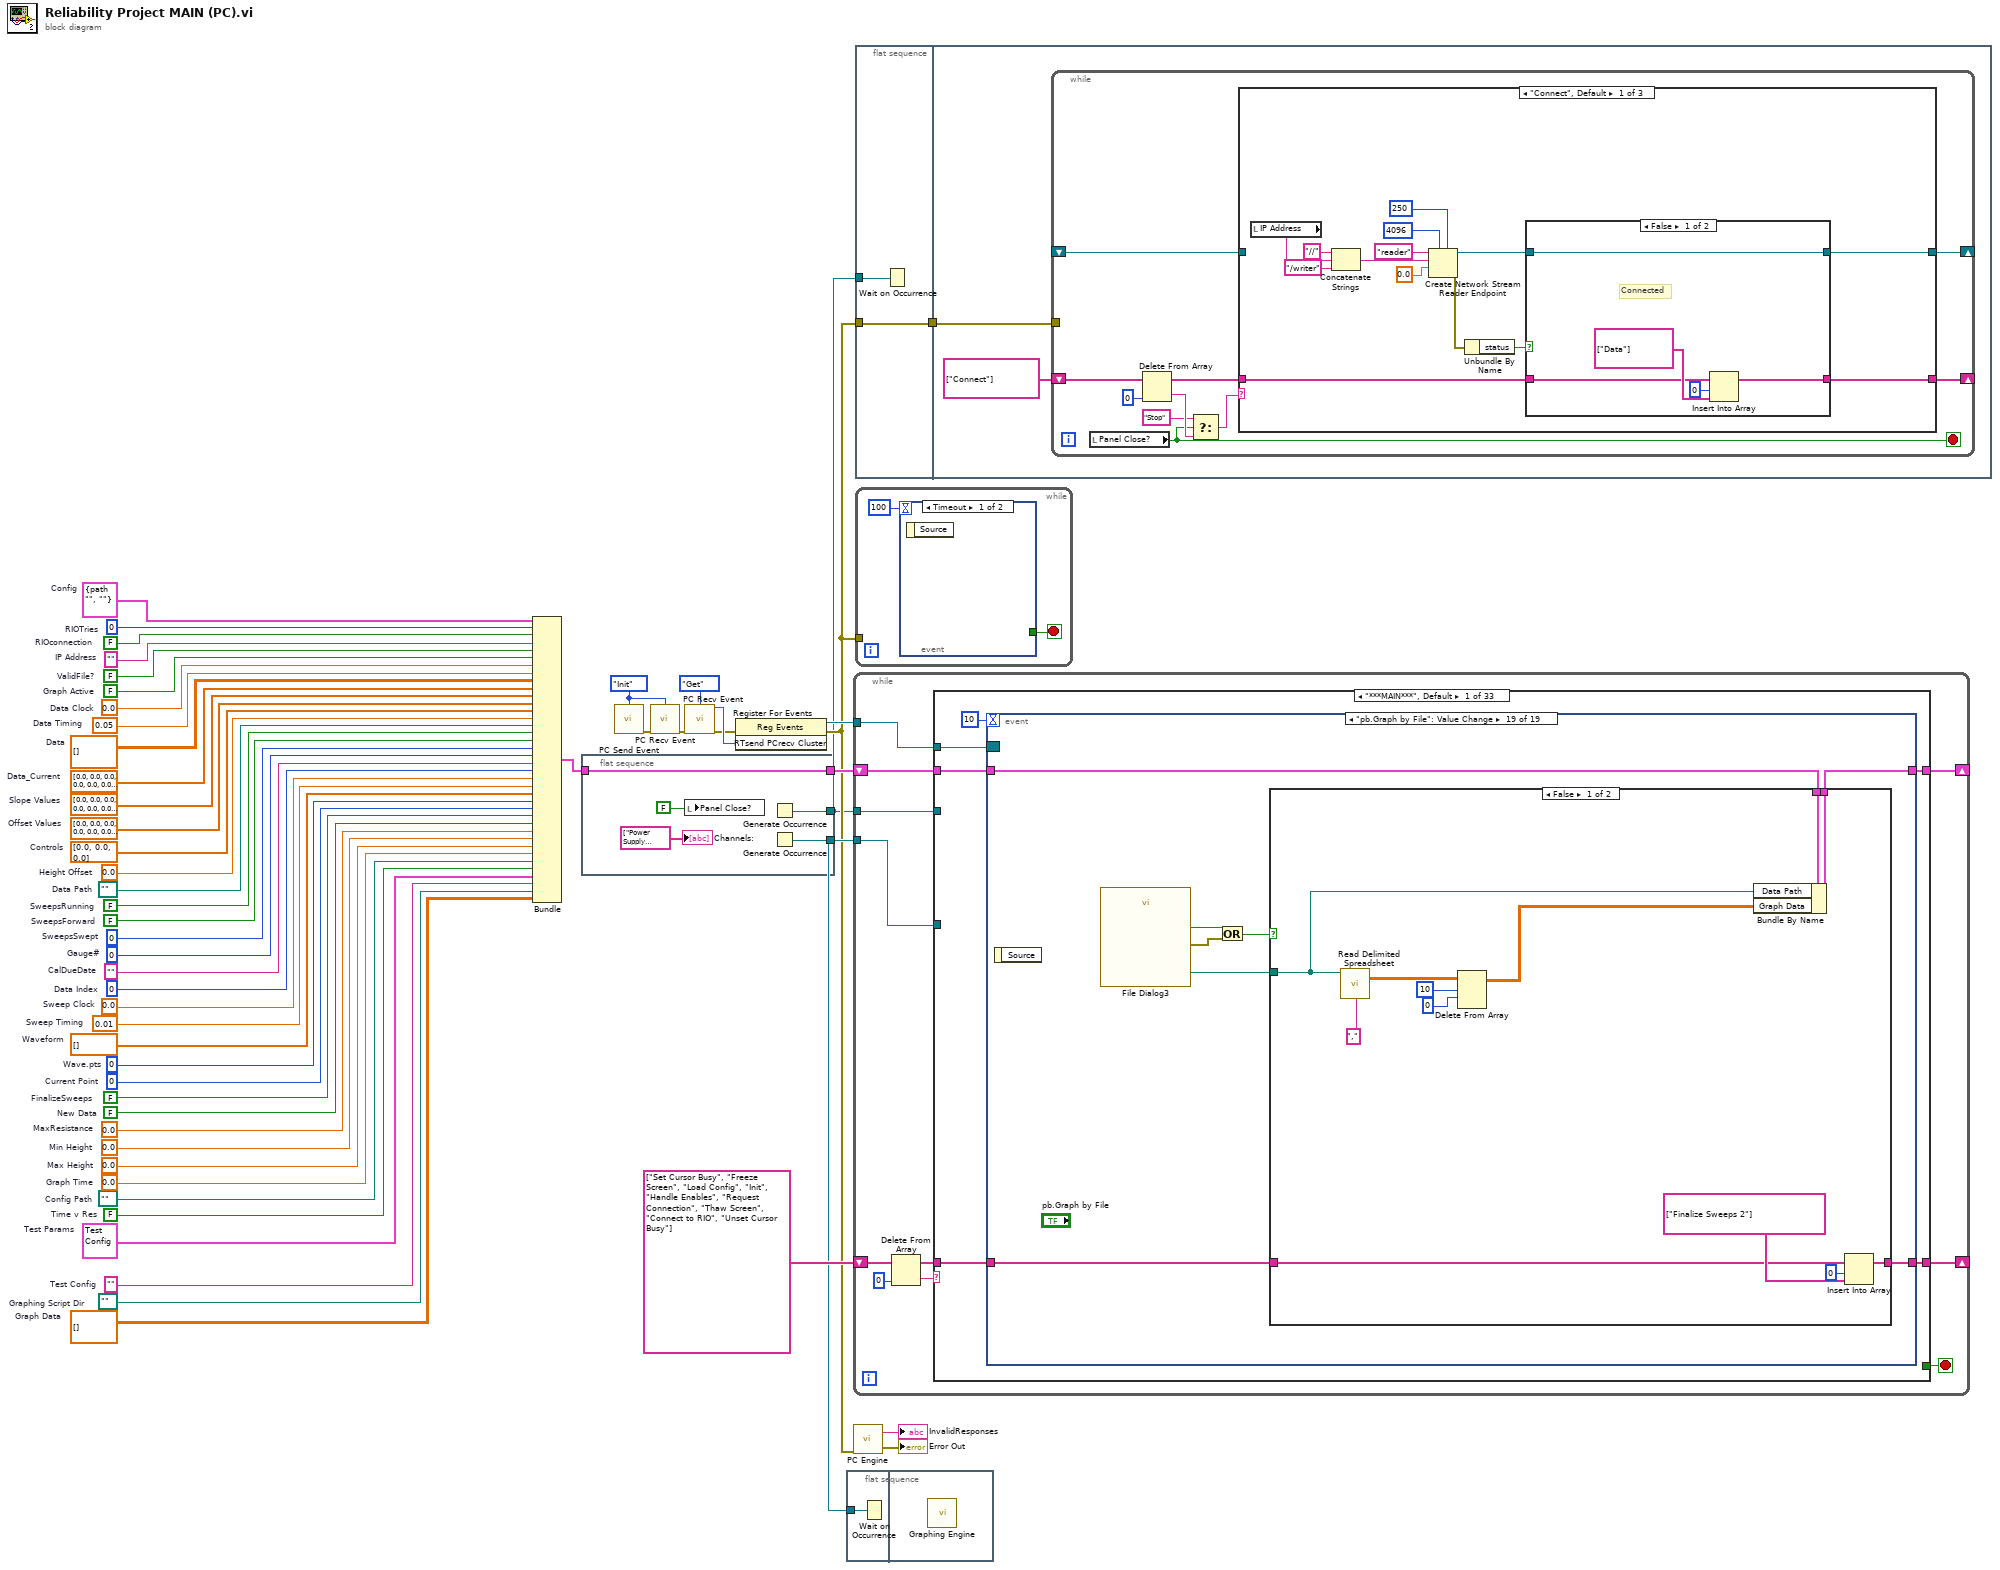
[diagram p0: block diagram]
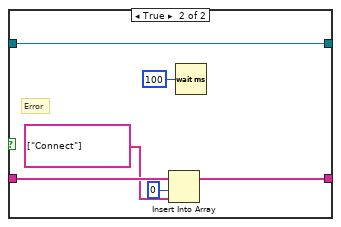
[diagram p2: hidden frame]
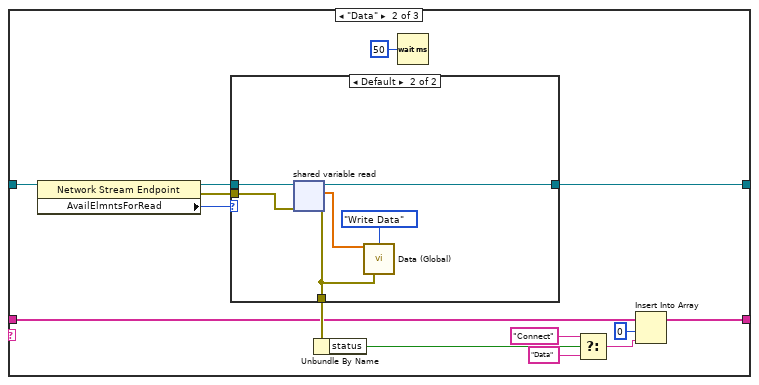
[diagram p3: hidden frame]
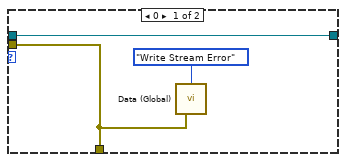
[diagram p4: hidden frame]
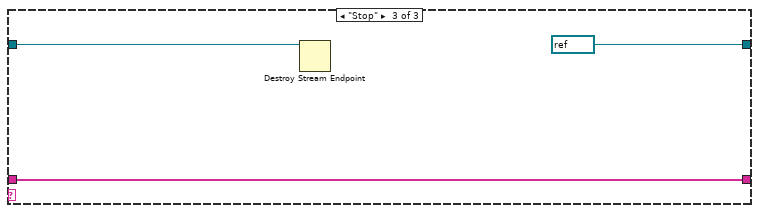
[diagram p5: hidden frame]
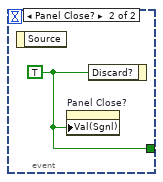
[diagram p6: hidden frame]
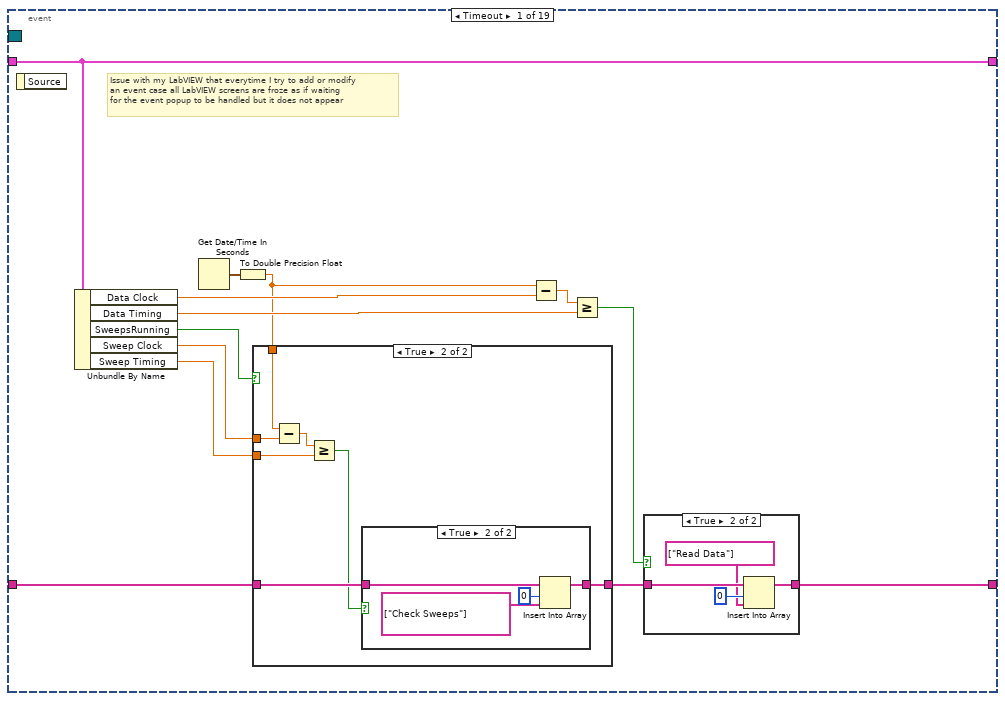
[diagram p7: hidden frame]
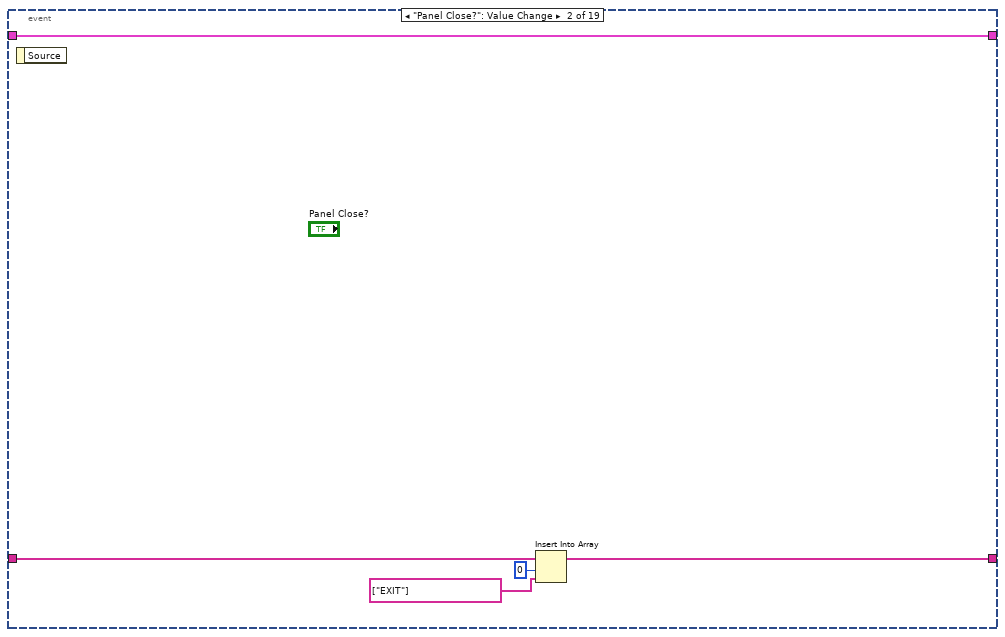
[diagram p11: hidden frame]
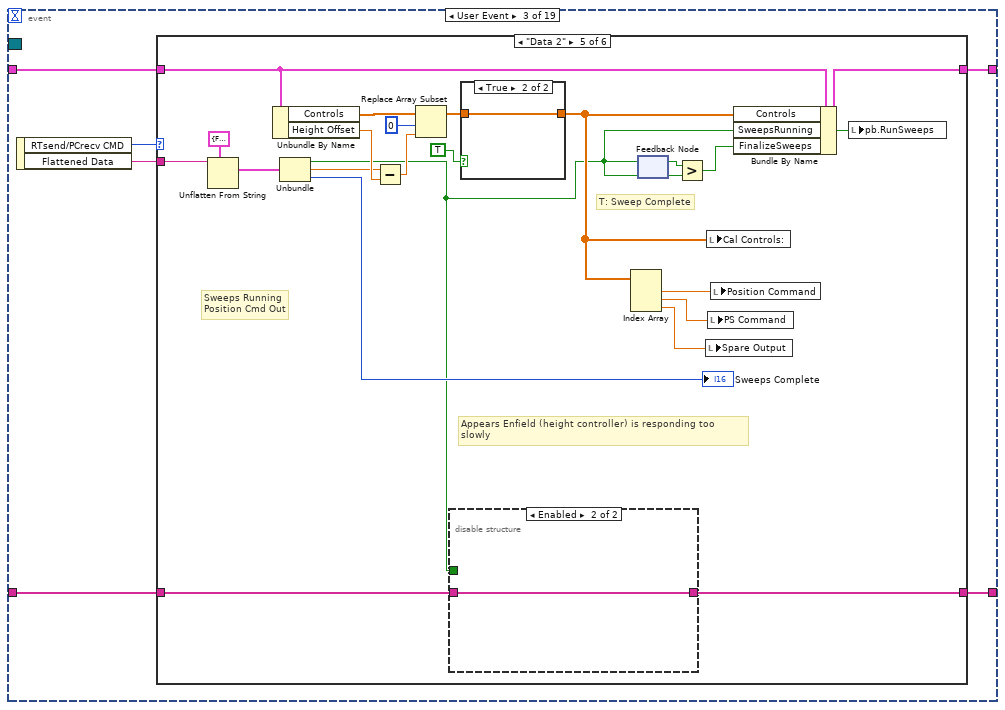
[diagram p12: hidden frame]
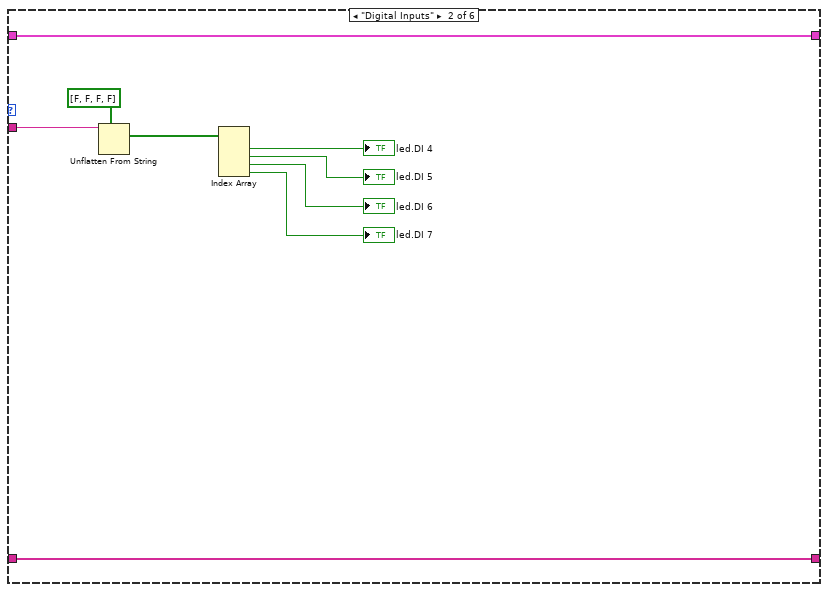
[diagram p14: hidden frame]
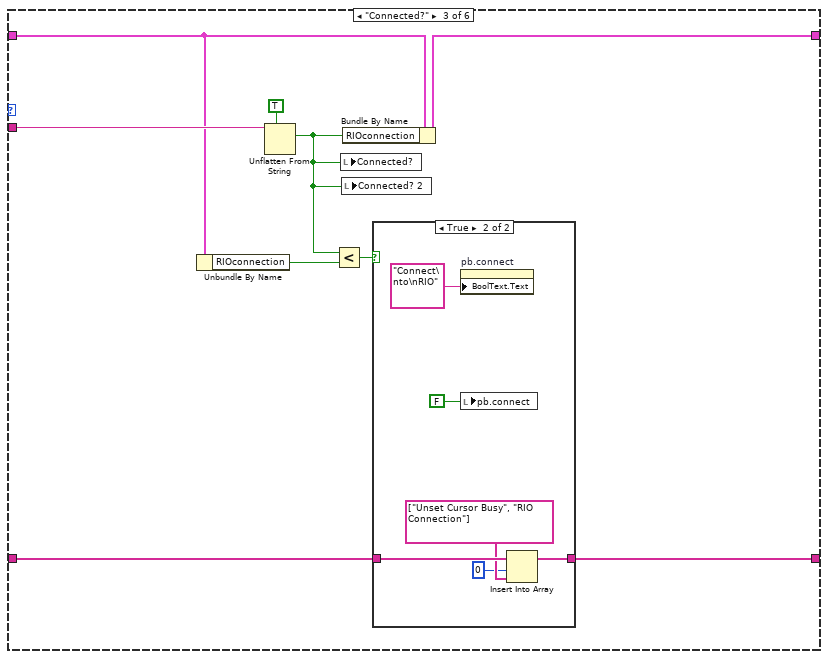
[diagram p15: hidden frame]
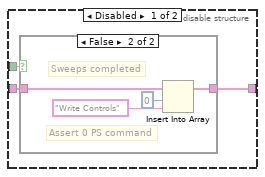
[diagram p18: hidden frame]
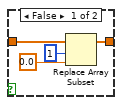
[diagram p20: hidden frame]
diagram:
  w1 = dbl[][] []  # Graph Data
  w2 = path ""  # Graphing Script Dir
  w3 = ""  # Test Config
  w4 = T8 {"Test Header"={"CA Number:"="", "Part Model:"="", "Part Serial Number:"="", "Technician Name:"="", "Test Fluid:"="", "Hours Description:"="", "Data Storage Folder:"=path ""}, "Test Style"=enum."Wet Test", "Bias Resistance"=nan, "Height Offset"=nan, "Graph Parameters"={"Tol Path"=path "C:/Users/gtetil/Documents/Projects/Reliability-Sweeper/Source/Files/Graphing Script/E7x Tolerance (MS, dry).csv", "Tol Band Color"=enum."Red", "Graph Type"=enum."H vs R & T vs R (1 Cycle)", "Height Min"=-15, "Height Max"=250, "Height Interval"=50, "Res Max"=1250, "Res Interval"=100, "Time Max"=10, "Time Interval"=1, "Graph Output File"=enum."pdf", "Auto Open"=TRUE}, "Test Parameters"={"Sweep Start Height"=0.0, "Sweep End Height"=0.0, "Sweep Time (s)"=0.0, "Sweep PS Cmd"=0.0, "Number of Sweeps"=0}}  # Test Params
  w5 = FALSE  # Time v Res
  w6 = path ""  # Config Path
  w7 = T10 {"Test Config Path"=path "", "RT IP Address"=""}  # Config
  w8 = 0.0  # Graph Time
  w13 = 0.0  # Max Height
  w14 = 0.0  # Min Height
  w15 = 0.0  # MaxResistance
  w16 = FALSE  # New Data
  w17 = FALSE  # FinalizeSweeps
  w20 = 0  # Current Point
  w19 = 0  # Wave.pts
  w18 = dbl[] []  # Waveform
  w21 = 0.01  # Sweep Timing
  w22 = 0.0  # Sweep Clock
  w23 = 0  # Data Index
  w25 = 0  # Gauge#
  w24 = ""  # CalDueDate
  w26 = dbl[] [0.0, 0.0, 0.0, 0.0, 0.0, 0.0, 0.0]  # Data_Current
  w28 = 0  # SweepsSwept
  w29 = FALSE  # SweepsForward
  w30 = FALSE  # SweepsRunning
  w31 = path ""  # Data Path
  w32 = 0.0  # Height Offset
  w33 = dbl[] [0.0, 0.0, 0.0]  # Controls
  w27 = dbl[] [0.0, 0.0, 0.0, 0.0, 0.0, 0.0, 0.0]  # Slope Values
  w34 = dbl[] [0.0, 0.0, 0.0, 0.0, 0.0, 0.0, 0.0]  # Offset Values
  w35 = dbl[][] []  # Data
  w36 = 0.05  # Data Timing
  w37 = 0.0  # Data Clock
  w38 = FALSE  # Graph Active
  w45 = Event_Mode."Init" ("Mode")
  w51 = FALSE  # ValidFile?
  w52 = ""  # IP Address
  w53 = 0  # RIOTries
  w54 = FALSE  # RIOconnection
  n1 = Bundle("Config"=w7, "RIOTries"=w53, "RIOconnection"=w54, "IP Address"=w52, "ValidFile?"=w51, "Graph Active"=w38, "Data Clock"=w37, "Data Timing"=w36, "Data"=w35, "Data_Current"=w26, "Slope Values"=w27, "Offset Values"=w34, "Controls"=w33, "Height Offset"=w32, "Data Path"=w31, "SweepsRunning"=w30, "SweepsForward"=w29, "SweepsSwept"=w28, "Gauge#"=w25, "CalDueDate"=w24, "Data Index"=w23, "Sweep Clock"=w22, "Sweep Timing"=w21, "Waveform"=w18, "Wave.pts"=w19, "Current Point"=w20, "FinalizeSweeps"=w17, "New Data"=w16, "MaxResistance"=w15, "Min Height"=w14, "Max Height"=w13, "Graph Time"=w8, "Config Path"=w6, "Time v Res"=w5, "Test Params"=w4, "Test Config"=w3, "Graphing Script Dir"=w2, "Graph Data"=w1) -> (w50:T12)  [unwired: 1 in]
  n2 = flat-sequence {
    tunnel: w50 -> [w59]
    tunnel: [w59] -> w42
    tunnel: [w56] -> w12
    tunnel: [w55] -> w9
    frame #0 {
      n3 = local write "Panel Close?"(FALSE ("Panel Close?")) -> ()
      n4 = Generate Occurrence() -> (w55:refnum<k4>)
      n5 = Generate Occurrence() -> (w56:refnum<k4>)
      "Channels:" <- string[] ["Power Supply Voltage", "Level Sender Voltage", "AI-3 Spare", "Height Gauge", "Position Command", "Power Supply Command", "Spare Output"] ("Channels")
    }
  }
  n6 = call "PC Send Event.vi"("Mode"=w45) -> ("Error Out"=w44:errorcluster)  [unwired: 13 in, 1 out]
  n7 = call "PC Recv Event.vi"("Mode"=w45, "Error In"=w44) -> ("Error Out"=w47:errorcluster)  [unwired: 12 in, 1 out]
  n8 = call "PC Recv Event.vi"("Mode"=Event_Mode."Get", "Error In"=w47) -> ("RTsend PCrecv Cluster"=w46:refnum<user-event>, "Error Out"=w43:errorcluster)  [unwired: 12 in]
  n9 = register-events(error in=w43, w46) -> (reference out=w49:refnum<event-registration>, error out=w11:errorcluster)  [unwired: 1 in]
  n10 = flat-sequence {
    tunnel: w12 -> [w60]
    frame #0 {
      n11 = Wait on Occurrence(2:w60) -> ()  [unwired: 2 in, 1 out]
    }
    frame #1 {
      n12 = call "Graphing Engine.vi"() -> ()  [unwired: 12 in]
    }
  }
  n13 = while {
    shift-right: [w68] -> _
    shift-left: string[] ["Set Cursor Busy", "Freeze Screen", "Load Config", "Init", "Handle Enables", "Request Connection", "Thaw Screen", "Connect to RIO", "Unset Cursor Busy"] -> [w71]
    shift-right: [w63] -> _
    shift-left: w42 -> [w67]
    tunnel: w49 -> [w65]
    tunnel: w12 -> [w62]
    tunnel: w9 -> [w61]
    stop <- w66 stop-if-true
    n14 = Delete From Array(array=w71, index=0) -> (deleted portion=w64:string, array with subset deleted=w69:string[])  [unwired: 1 in]
    n15 = case shown="\"***MAIN***\", Default" w64 {
      selector: w64 -> [_ _ _ _ _ _ _ _ _ _ _ _ _ _ _ _ _ _ _ _ _ _ _ _ _ _ _ _ _ w1422 _ _ _]
      tunnel: w69 -> [w74 w537 w562 w566 w588 w595 w668 w676 w698 w722 w730 w757 w771 w828 w866 w894 w900 w979 w1045 w1051 w1085 w1198 w1306 w1327 w1331 w1333 w1344 w1346 w1420 w1423 w1427 w1429 w1436]
      tunnel: [w72 w538 w562 w565 w585 w592 w667 w675 w697 w721 w729 w756 w770 w792 w866 w894 w900 w979 w1044 w1051 w1084 w1197 w1305 w1326 w1331 w1333 w1344 w1345 w1420 w1423 w1427 w1429 w1436] -> w68
      tunnel: w67 -> [w76 w536 w563 w574 w589 w597 w620 w672 w691 w712 w725 w737 w768 w831 w865 w893 w899 w970 w1043 w1050 w1087 w1204 w1297 w1323 w1332 w1334 w1343 w1348 w1406 w1424 w1428 w1430 w1437]
      tunnel: [_ FALSE _ _ _ _ _ _ _ _ _ _ _ _ _ _ _ _ _ _ _ _ _ _ _ _ _ _ _ _ _ _ TRUE] -> w66
      tunnel: w65 -> [w77 _ _ _ _ _ _ _ _ _ _ _ _ _ _ _ _ _ _ _ _ _ _ _ _ _ _ _ _ _ _ _ _]
      tunnel: [w75 w535 w563 w573 w589 w596 w620 w673 w692 w711 w724 w737 w768 w830 w865 w893 w899 w970 w1042 w1047 w1086 w1203 w1294 w1323 w1332 w1334 w1343 w1347 w1406 w1424 w1428 w1430 w1437] -> w63
      tunnel: w62 -> [_ w549 _ _ _ _ _ _ _ _ _ _ _ _ _ _ _ _ _ _ _ _ _ _ _ _ _ _ _ _ _ _ _]
      tunnel: w61 -> [_ w547 _ _ _ _ _ _ _ _ _ _ _ _ _ _ _ _ _ _ _ _ _ _ _ _ _ _ _ _ _ _ _]
      frame "***MAIN***", Default {
        n16 = event shown="[18] \"pb.Graph by File\": Value Change" {
          selector: w77 -> [_ _ _ _ _ _ _ _ _ _ _ _ _ _ _ _ _ _ _]
          dyn-events: _ -> [_ _ _ _ _ _ _ _ _ _ _ _ _ _ _ _ _ _ _]
          timeout: 10 -> [_ _ _ _ _ _ _ _ _ _ _ _ _ _ _ _ _ _ _]
          tunnel: [w79 w113 w115 w218 w235 w238 w255 w266 w280 w301 w305 w318 w353 w357 w466 w483 w502 w507 w511] -> w75
          tunnel: w76 -> [w79 w113 w117 w219 w235 w239 w255 w266 w281 w302 w305 w318 w354 w358 w467 w484 w502 w507 w512]
          tunnel: w74 -> [w84 w112 w116 w216 w234 w237 w251 w268 w273 w300 w304 w308 w346 w359 w472 w488 w499 w504 w515]
          tunnel: [w78 w109 w114 w214 w234 w237 w250 w267 w272 w299 w304 w307 w345 w356 w471 w487 w498 w503 w514] -> w72
          event Timeout {
            # "Issue with my LabVIEW that everytime I try to add or modify\nan event case all LabVIEW screens are froze as if waiting\nfor the event popup to be handled but it does not appear"
            n17 = event-data() -> ()  [unwired: 1 in, 1 out]
            n18 = Unbundle By Name(w79) -> ("Data Clock"=w90:dbl, "Data Timing"=w89:dbl, "SweepsRunning"=w85:bool, "Sweep Clock"=w82:dbl, "Sweep Timing"=w81:dbl)
            n19 = Get Date/Time In Seconds() -> (seconds since 1Jan1904=w87:timestamp)
            n20 = To Double Precision Float(number=w87) -> (double precision float=w83:dbl)
            n21 = case shown="True" w85 {
              tunnel: w84 -> [w91 w94]
              tunnel: w83 -> [_ w97]
              tunnel: w82 -> [_ w96]
              tunnel: w81 -> [_ w95]
              tunnel: [w91 w93] -> w80
              frame False {
              }
              frame True {
                n22 = Subtract(x=w97, y=w96) -> (x-y=w98:dbl)
                n23 = Greater Or Equal?(x=w98, y=w95) -> (x >= y?=w92:bool)
                n24 = case shown="True" w92 {
                  tunnel: w94 -> [w99 w101]
                  tunnel: [w99 w100] -> w93
                  frame False {
                  }
                  frame True {
                    n25 = Insert Into Array(array=w101, index=0, new element=string[] ["Check Sweeps"]) -> (w100:string[])
                  }
                }
              }
            }
            n26 = Subtract(x=w83, y=w90) -> (x-y=w86:dbl)
            n27 = Greater Or Equal?(x=w86, y=w89) -> (x >= y?=w88:bool)
            n28 = case shown="True" w88 {
              tunnel: w80 -> [w104 w108]
              tunnel: [w104 w107] -> w78
              frame False {
              }
              frame True {
                n29 = Insert Into Array(array=w108, index=0, new element=string[] ["Read Data"]) -> (w107:string[])
              }
            }
          }
          event "Panel Close?": Value Change {
            n30 = event-data() -> ()  [unwired: 1 in, 1 out]
            n31 = Insert Into Array(array=w112, index=0, new element=string[] ["EXIT"]) -> (w109:string[])
          }
          event User Event {
            n32 = event-data() -> ("RTsend/PCrecv CMD"=w119:T22, "Flattened Data"=w118:string)  [unwired: 1 in]
            n33 = case shown="\"Data 2\"" w119 {
              tunnel: w118 -> [_ w130 w139 _ w170 w212]
              tunnel: w117 -> [w121 w128 w136 w148 w166 w209]
              tunnel: w116 -> [w120 w129 w134 w147 w152 w188]
              tunnel: [w121 w128 w137 w148 w167 w210] -> w115
              tunnel: [w120 w129 w131 w147 w151 w187] -> w114
              frame Default {
              }
              frame "Digital Inputs" {
                n34 = Unflatten From String(type=bool[] [FALSE, FALSE, FALSE, FALSE], binary string=w130) -> (value=w126:bool[])  [unwired: 3 in, 2 out]
                n35 = Index Array(array=w126) -> (element #1=→"led.DI 4":bool, element #2=→"led.DI 5":bool, element #3=→"led.DI 6":bool, element #4=→"led.DI 7":bool)  [unwired: 4 in]
              }
              frame "Connected?" {
                n36 = Unbundle By Name(w136) -> ("RIOconnection"=w132:bool)
                n37 = Unflatten From String(type=TRUE, binary string=w139) -> (value=w133:bool)  [unwired: 3 in, 2 out]
                n38 = Less?(x=w133, y=w132) -> (x < y?=w135:bool)
                n39 = local write "Connected?"(w133) -> ()
                n40 = local write "Connected? 2"(w133) -> ()
                n41 = Bundle By Name(cluster=w136, "RIOconnection"=w133) -> (w137:T12)
                n42 = case shown="True" w135 {
                  tunnel: w134 -> [w140 w146]
                  tunnel: [w140 w145] -> w131
                  frame False {
                  }
                  frame True {
                    n43 = property on="pb.connect" class="Bool (strict)"("BoolText.Text"="Connect\nto\nRIO" ("Boolean Text.Text")) -> ()  [unwired: 2 in, 2 out]
                    n44 = local write "pb.connect"(FALSE ("pb.RetryRIO")) -> ()
                    n45 = Insert Into Array(array=w146, index=0, new element=string[] ["Unset Cursor Busy", "RIO Connection"]) -> (w145:string[])
                  }
                }
              }
              frame "Data" {
                # "No longer using this connection to stream the data"
              }
              frame "Data 2" {
                # "Appears Enfield (height controller) is responding too slowly"
                # "T: Sweep Complete"
                # "Sweeps Running\nPosition Cmd Out"
                n46 = Unflatten From String(type=cluster{bool, dbl, i16} {FALSE, 0.0, 0}, binary string=w170) -> (value=w168:cluster{bool, dbl, i16})  [unwired: 3 in, 2 out]
                n47 = Unbundle By Name(w166) -> ("Controls"=w165:dbl[], "Height Offset"=w158:dbl)
                n48 = Unbundle(w168) -> (w150:bool, w157:dbl, →"Sweeps Complete":i16)
                n49 = Subtract(x=w157, y=w158) -> (x-y=w156:dbl)
                n50 = Replace Array Subset(array=w165, new element=w156, index=0) -> (w154:dbl[])
                n51 = disable-structure shown="Enabled" {
                  disable-tunnel: w152 -> [w173 w179]
                  disable-tunnel: [w172 w179] -> w151
                  disable-tunnel: w150 -> [w171 _]
                  frame Disabled {
                    n52 = case shown="False" w171 {
                      tunnel: w173 -> [w174 w178]
                      tunnel: [w174 w177] -> w172
                      frame True {
                        # "Do not interrupt"
                        # "Sweeps running"
                      }
                      frame False {
                        # "Assert 0 PS command"
                        # "Sweeps completed"
                        n53 = Insert Into Array(array=w178, index=0, new element="Write Controls" ("new element/subarray")) -> (w177:string[])
                      }
                    }
                  }
                  frame Enabled {
                  }
                }
                n54 = case shown="True" TRUE {
                  tunnel: w154 -> [w183 w184]
                  tunnel: [w182 w184] -> w153
                  frame False {
                    n55 = Replace Array Subset(array=w183, new element=0.0 ("new element/subarray"), index=1) -> (w182:dbl[])
                  }
                  frame True {
                  }
                }
                n56 = Index Array(array=w153) -> (element #1=w163:dbl, element #2=w162:dbl, element #3=w161:dbl)  [unwired: 3 in]
                n57 = feedback-in #1(w150) -> ()
                n58 = feedback #1(w150) -> (w160:bool)
                n59 = Greater?(x=w160, y=w150) -> (0:w159:bool)
                n60 = local write "Spare Output"(w161) -> ()
                n61 = local write "Cal Controls:"(w153) -> ()
                n62 = local write "PS Command"(w162) -> ()
                n63 = local write "Position Command"(w163) -> ()
                n64 = Bundle By Name(cluster=w166, "Controls"=w153, "SweepsRunning"=w150, "FinalizeSweeps"=w159) -> (w167:T12)
                n65 = local write "pb.RunSweeps"(w150) -> ()
              }
              frame "Cal2PC" {
                w197 = "/" ("regular expression")
                # "?? add 2000"
                n66 = Unflatten From String(type=cluster{dbl[], dbl[], i32, string} {[], [], 0, ""}, binary string=w212) -> (value=w211:cluster{dbl[], dbl[], i32, string})  [unwired: 3 in, 2 out]
                n67 = Unbundle(w211) -> (w206:dbl[], w205:dbl[], w204:i32, w193:string)
                n68 = Match Pattern(string=w193, regular expression=w197) -> (before substring=w196:string, after substring=w198:string)  [unwired: 1 in, 2 out]
                n69 = Match Pattern(string=w198, regular expression=w197) -> (before substring=w195:string, after substring=w194:string)  [unwired: 1 in, 2 out]
                n70 = call "Data (Global).vi"("Mode"=enum16{"Read Data", "Write Data", "Write Cal"}."Write Cal", "Slope"=w206, "Offset"=w205) -> ()  [unwired: 9 in, 4 out]
                n71 = Decimal String To Number(string=w195) -> (number=w200:i32)  [unwired: 2 in, 1 out]
                n72 = Decimal String To Number(string=w196) -> (number=w199:i32)  [unwired: 2 in, 1 out]
                n73 = Decimal String To Number(string=w194) -> (number=w191:i32)  [unwired: 2 in, 1 out]
                n74 = Bundle By Name(cluster=w209, "Slope Values"=w206, "Offset Values"=w205, "Gauge#"=w204, "CalDueDate"=w193) -> (w210:T12)
                n75 = Add(x=w191, y=2000) -> (x+y=w190:i32)
                n76 = Bundle By Name(cluster=T13 {"fractional second"=0.0, "second"=0, "minute"=0, "hour"=0, "day of month"=0, "month"=0, "year"=0, "day of week"=0, "day of year"=0, "DST"=0} ("date time rec"), "day of month"=w200, "month"=w199, "year"=w190) -> (w201:T13)
                n77 = Insert Into Array(array=w188, index=0, new element="Write Controls" ("new element/subarray")) -> (w187:string[])
                n78 = Build Array(w204) -> (w203:i32[])
                n79 = Date/Time To Seconds(2:w201) -> (0:w192:timestamp)  [unwired: 1 in]
                n80 = local write "Slope Values:"(w206) -> ()
                n81 = local write "Offset Values:"(w205) -> ()
                n82 = local write "Cal Due Date:"(w192) -> ()
                n83 = local write "Gauge Number:"(w203) -> ()
              }
            }
          }
          event "Position Command", "PS Command", "Spare Output": Value Change {
            n84 = event-data() -> ()  [unwired: 1 in, 1 out]
            n85 = Build Array("Position Command", "PS Command", "Spare Output") -> (w217:dbl[])
            n86 = Insert Into Array(array=w216, index=0, new element="Write Controls" ("new element/subarray")) -> (w214:string[])
            n87 = Bundle By Name(cluster=w219, "Controls"=w217) -> (w218:T12)
            n88 = local write "Cal Controls:"(w217) -> ()
          }
          event "pb.DO0", "pb.DO1", "pb.DO2", "pb.DO3": Value Change {
            n89 = event-data() -> ()  [unwired: 1 in, 1 out]
            n90 = Build Array("pb.DO0", "pb.DO1", "pb.DO2", "pb.DO3") -> (w227:bool[])
            n91 = Flatten To String(anything=w227) -> (data string=w225:string)  [unwired: 3 in, 2 out]
            n92 = Bundle("Digital Outputs", "data string"=w225) -> (w224:cluster{string, "data string":string})  [unwired: 1 in]
            n93 = Flatten To String(anything=w224) -> (data string=w223:string)  [unwired: 3 in, 2 out]
            n94 = call "PC Send Event.vi"("PC Send Command"=PCsend_RTrecv_CMD."Digital Outputs", "Mode"=Event_Mode."Set", "Flattened Data"=w223) -> ()  [unwired: 11 in, 2 out]
          }
          event "pb.graph control": Value Change {
            n95 = event-data() -> ()  [unwired: 1 in, 1 out]
            n96 = case shown="True" "pb.graph control" {
              frame False {
              }
              frame True {
                n97 = property on="Chart" class="WFChart (strict)"("History Data"=dbl[][] []) -> ()  [unwired: 2 in, 2 out]
              }
            }
            n98 = Bundle By Name(cluster=w239, "Graph Active"="pb.graph control") -> (w238:T12)
          }
          event "pb.RevertCal": Value Change {
            n99 = event-data() -> ()  [unwired: 1 in, 6 out]
            n100 = Unbundle By Name(w255) -> ("Slope Values"=w242:dbl[], "Offset Values"=w241:dbl[])
            n101 = local write "Offset Values:"(w241) -> ()
            n102 = local write "Slope Values:"(w242) -> ()
            n103 = Bundle("Slope Values"=w242, "Offset Values"=w241) -> (w243:T23)  [unwired: 1 in]
            n104 = call "Data (Global).vi"("Mode"=enum16{"Read Data", "Write Data", "Write Cal"}."Write Cal", "Slope"=w242, "Offset"=w241) -> ()  [unwired: 9 in, 4 out]
            n105 = Insert Into Array(array=w251, index=0, new element="Write Controls" ("new element/subarray")) -> (w250:string[])
            n106 = Flatten To String(anything=w243) -> (data string=w246:string)  [unwired: 3 in, 2 out]
            n107 = Bundle("Cal2RT", "data string"=w246) -> (w245:cluster{string, "data string":string})  [unwired: 1 in]
            n108 = Flatten To String(anything=w245) -> (data string=w244:string)  [unwired: 3 in, 2 out]
            n109 = call "PC Send Event.vi"("PC Send Command"=PCsend_RTrecv_CMD."Cal2RT", "Mode"=Event_Mode."Set", "Flattened Data"=w244) -> ()  [unwired: 11 in, 2 out]
          }
          event "Offset Values:", "Slope Values:": Value Change {
            n110 = event-data() -> ()  [unwired: 1 in, 6 out]
            n111 = call "Data (Global).vi"("Mode"=enum16{"Read Data", "Write Data", "Write Cal"}."Write Cal", "Slope"="Slope Values:", "Offset"="Offset Values:") -> ()  [unwired: 9 in, 4 out]
            n112 = Bundle By Name(cluster=cluster{"Slope":dbl[], "Offset":dbl[]} {"Slope"=[], "Offset"=[]}, "Slope"="Slope Values:", "Offset"="Offset Values:") -> (w258:cluster{"Slope":dbl[], "Offset":dbl[]})
            n113 = Flatten To String(anything=w258) -> (data string=w262:string)  [unwired: 3 in, 2 out]
            n114 = Insert Into Array(array=w268, index=0, new element="Write Controls" ("new element/subarray")) -> (w267:string[])
            n115 = Bundle("Cal2RT", "data string"=w262) -> (w261:cluster{string, "data string":string})  [unwired: 1 in]
            n116 = Flatten To String(anything=w261) -> (data string=w260:string)  [unwired: 3 in, 2 out]
            n117 = call "PC Send Event.vi"("PC Send Command"=PCsend_RTrecv_CMD."Cal2RT", "Mode"=Event_Mode."Set", "Flattened Data"=w260) -> ()  [unwired: 11 in, 2 out]
          }
          event "Cal Controls:": Value Change {
            n118 = event-data() -> ()  [unwired: 1 in, 1 out]
            n119 = Index Array(array="Cal Controls:") -> (element #1=w278:dbl, element #2=w277:dbl, element #3=w276:dbl)  [unwired: 3 in]
            n120 = local write "Spare Output"(w276) -> ()
            n121 = local write "PS Command"(w277) -> ()
            n122 = local write "Position Command"(w278) -> ()
            n123 = Insert Into Array(array=w273, index=0, new element="Write Controls" ("new element/subarray")) -> (w272:string[])
            n124 = Bundle By Name(cluster=w281, "Controls"="Cal Controls:") -> (w280:T12)
          }
          event "pb.SaveCal": Value Change {
            n125 = event-data() -> ()  [unwired: 1 in, 1 out]
            n126 = local read "Offset Values:"() -> (w296:dbl[])
            n127 = local read "Slope Values:"() -> (w297:dbl[])
            n128 = Index Array(array="Gauge Number:", index=0) -> (element=w283:i32)
            n129 = Format Date/Time String(time format string (%c)="%m/%d/%y", seconds (now)="Cal Due Date:") -> (date/time string=w282:string)  [unwired: 1 in]
            n130 = Bundle By Name(cluster=w302, "Slope Values"=w297, "Offset Values"=w296, "Gauge#"=w283, "CalDueDate"=w282) -> (w301:T12)
            n131 = Bundle("Numeric"=w283, "date/time string"=w282) -> (w284:T24)  [unwired: 1 in]
            n132 = Insert Into Array(array=w300, index=0, new element="Save Cal" ("new element/subarray")) -> (w299:string[])
            n133 = Flatten To String(anything=w284) -> (data string=w287:string)  [unwired: 3 in, 2 out]
            n134 = Bundle("Save Cal", "data string"=w287) -> (w286:cluster{string, "data string":string})  [unwired: 1 in]
            n135 = Flatten To String(anything=w286) -> (data string=w285:string)  [unwired: 3 in, 2 out]
            n136 = call "PC Send Event.vi"("PC Send Command"=PCsend_RTrecv_CMD."Save Cal", "Mode"=Event_Mode."Set", "Flattened Data"=w285) -> ()  [unwired: 11 in, 2 out]
          }
          event "pb.CalPage": Value Change {
            n137 = event-data() -> ()  [unwired: 1 in, 1 out]
            n138 = local write "Screen"(T15."Calibration" ("Screen")) -> ()
          }
          event "pb.RunScreen": Value Change {
            n139 = event-data() -> ()  [unwired: 1 in, 1 out]
            n140 = Unbundle By Name(w318) -> ("Slope Values"=w310:dbl[], "Offset Values"=w309:dbl[])
            n141 = local read "Offset Values:"() -> (w316:dbl[])
            n142 = local read "Slope Values:"() -> (w317:dbl[])
            n143 = Equal?(x=w317, y=w310) -> (x = y?=w314:bool[])
            n144 = Equal?(x=w309, y=w316) -> (x = y?=w315:bool[])
            n145 = And Array Elements(Boolean array=w314) -> (logical AND=w313:bool)
            n146 = And Array Elements(Boolean array=w315) -> (logical AND=w312:bool)
            n147 = And(x=w313, y=w312) -> (x .and. y?=w311:bool)
            n148 = flat-sequence {
              tunnel: w311 -> [w323]
              tunnel: w310 -> [w322]
              tunnel: w309 -> [w321]
              tunnel: w308 -> [w320]
              tunnel: [w319] -> w306
              tunnel: [w340] -> w307
              tunnel: w306 -> [w340]
              frame #0 {
                n149 = case shown="False" w323 {
                  tunnel: w322 -> [w325 _]
                  tunnel: w321 -> [w324 _]
                  tunnel: w320 -> [w334 w338]
                  tunnel: [w333 w338] -> w319
                  frame False {
                    # "Mismatched Values\n-\nRevert to previous values"
                    n150 = Bundle("Slope Values"=w325, "Offset Values"=w324) -> (w326:T23)  [unwired: 1 in]
                    n151 = local write "Offset Values:"(w324) -> ()
                    n152 = local write "Slope Values:"(w325) -> ()
                    n153 = call "Data (Global).vi"("Mode"=enum16{"Read Data", "Write Data", "Write Cal"}."Write Cal", "Slope"=w325, "Offset"=w324) -> ()  [unwired: 9 in, 4 out]
                    n154 = Flatten To String(anything=w326) -> (data string=w329:string)  [unwired: 3 in, 2 out]
                    n155 = Bundle("Cal2RT", "data string"=w329) -> (w328:cluster{string, "data string":string})  [unwired: 1 in]
                    n156 = Flatten To String(anything=w328) -> (data string=w327:string)  [unwired: 3 in, 2 out]
                    n157 = Insert Into Array(array=w334, index=0, new element="Write Controls" ("new element/subarray")) -> (w333:string[])
                    n158 = call "PC Send Event.vi"("PC Send Command"=PCsend_RTrecv_CMD."Cal2RT", "Mode"=Event_Mode."Set", "Flattened Data"=w327) -> ()  [unwired: 11 in, 2 out]
                  }
                  frame True {
                    # "Values Match\n-\nContinue"
                  }
                }
              }
              frame #1 {
                n159 = local write "Screen"(T15."Run Screen" ("Screen")) -> ()
              }
            }
          }
          event "pb.TareHeight": Value Change {
            w342 = 0.0 ("new element/subarray")
            n160 = event-data() -> ()  [unwired: 1 in, 1 out]
            n161 = Unbundle By Name(w354) -> ("Data"=w352:dbl[][], "Controls"=w348:dbl[])
            n162 = Replace Array Subset(array=w348, new element=w342, index=0) -> (w343:dbl[])
            n163 = Index Array(array=w352, index (row)=0 ("disabled index (col)"), index (col)=3 ("disabled index (row)")) -> (element=w351:dbl)
            n164 = Bundle By Name(cluster=w354, "Height Offset"=w351, "Controls"=w343) -> (w353:T12)
            n165 = local write "Cal Controls:"(w343) -> ()
            n166 = local write "Relative Height"(w342) -> ()
            n167 = local write "Position Command"(w342) -> ()
            n168 = Insert Into Array(array=w346, index=0, new element=string[] ["Write Controls", "Save Test Config"]) -> (w345:string[])
          }
          event "pb.RunSweeps": Value Change {
            n169 = event-data() -> ()  [unwired: 1 in, 1 out]
            n170 = case shown="False" "pb.RunSweeps" {
              tunnel: w359 -> [w370 w396]
              tunnel: w358 -> [w368 w401]
              tunnel: w358 -> [w367 w398]
              tunnel: [w366 w397] -> w357
              tunnel: [w369 w395] -> w356
              frame False {
                w379 = 0.0 ("new element/subarray")
                # "Set power supply and spare to zero"
                # "Stop Sweeps"
                n171 = Unbundle By Name(w368) -> ("Controls"=w376:dbl[])
                n172 = call <vilib>:"Application Directory.vi"() -> ("Application Directory"=w364:path)
                n173 = Build Path(base path=w364, name or relative path="Temp") -> (appended path=w362:path)
                n174 = property on="pb.graph control" class="Bool (strict)"("Val(Sgnl)"=FALSE ("Value (Signaling)")) -> ()  [unwired: 2 in, 2 out]
                n175 = List Folder(path=w362) -> (path out=w361:path, filenames=w360:string[])  [unwired: 3 in, 2 out]
                n176 = for {
                  tunnel: w361 -> [w391]
                  tunnel: w360 -> [w390] mode=indexing
                  n177 = Build Path(base path=w391, name or relative path=w390) -> (appended path=w389:path)
                  n178 = Delete(path (use dialog)=w389) -> ()  [unwired: 4 in, 3 out]
                }
                n179 = Replace Array Subset(array=w376, new element #1=w379, index #1=1 ("index"), new element #2=w379, index #2=2 ("index")) -> (w380:dbl[])
                n180 = Index Array(array=w380) -> (element #1=w371:dbl, element #2=w372:dbl, element #3=w373:dbl)  [unwired: 3 in]
                n181 = Insert Into Array(array=w370, index=0, new element=string[] ["Write Controls", "Handle Enables"]) -> (w369:string[])
                n182 = local write "Spare Output"(w373) -> ()
                n183 = local write "PS Command"(w372) -> ()
                n184 = local write "Cal Controls:"(w380) -> ()
                n185 = local write "Position Command"(w371) -> ()
                n186 = Flatten To String(anything=FALSE) -> (data string=w383:string)  [unwired: 3 in, 2 out]
                n187 = Bundle("Start Sweep", "data string"=w383) -> (w382:cluster{string, "data string":string})  [unwired: 1 in]
                n188 = Flatten To String(anything=w382) -> (data string=w381:string)  [unwired: 3 in, 2 out]
                n189 = Bundle By Name(cluster=w367, "SweepsRunning"=FALSE, "Controls"=w380) -> (w366:T12)
                n190 = call "PC Send Event.vi"("PC Send Command"=PCsend_RTrecv_CMD."Start Sweep", "Mode"=Event_Mode."Set", "Flattened Data"=w381) -> ()  [unwired: 11 in, 2 out]
              }
              frame True {
                n191 = Unbundle By Name(w401) -> ("Test Params.Test Header.Data Storage Folder:"=w400:path, "Test Params.Test Header.Part Serial Number:"=w394:string)
                n192 = Empty String/Path?(string/path=w394) -> (empty?=w399:bool)
                n193 = case shown="False" w399 {
                  tunnel: w400 -> [w418 w433]
                  tunnel: w394 -> [w416 _]
                  tunnel: [w412 w430] -> w393
                  frame False {
                    # "SN exists"
                    n194 = Concatenate Strings(w416, ".csv" ("pattern")) -> (w408:string)
                    n195 = Build Path(base path=w418, name or relative path=w408) -> (appended path=w415:path)
                    n196 = call <vilib>:"Check if File or Folder Exists.vi"("path"=w415) -> ("file or folder exists?"=w414:bool, "dup path"=w413:path)  [unwired: 8 in, 1 out]
                    n197 = case shown="True" w414 {
                      tunnel: w413 -> [w419 w423]
                      tunnel: [w419 w422] -> w412
                      tunnel: "File exists, replace?" -> [_ w426]
                      tunnel: "Yes" -> [_ w425]
                      tunnel: "No" -> [_ w424]
                      frame False {
                        # "New SN - Continue"
                      }
                      frame True {
                        # "Used SN - Check"
                        n198 = Two Button Dialog(message=w426, 1:w424, 2:w425) -> (T button?=w421:bool)
                        n199 = Select(t=w423, s=w421, f=path "") -> (s? t:f=w422:path)
                      }
                    }
                  }
                  frame True {
                    # "SN DNE"
                    n200 = List Folder(path=w433, pattern="*.csv") -> (path out=w429:path, filenames=w432:string[])  [unwired: 2 in, 2 out]
                    n201 = while {
                      tunnel: w432 -> [w438]
                      tunnel: ".csv" ("pattern") -> [w445]
                      tunnel: [w434] -> w427
                      i -> [w450]
                      stop <- w447 stop-if-true
                      n202 = Increment(x=w450) -> (x+1=w439:i32)
                      n203 = Number To Decimal String(number=w439, width (-)=i16 4) -> (decimal integer string=w443:string)
                      n204 = Greater Or Equal?(x=w439, y=9999) -> (x >= y?=w448:bool)
                      n205 = call <vilib>:"Space Constant.vi"() -> ("String"=w440:string)
                      n206 = Search and Replace String(replace all?=TRUE ("replace all? (F)"), input string=w443, search string=w440, replace string="0" ("replace string (\"\")")) -> (result string=w437:string)  [unwired: 4 in, 3 out]
                      n207 = Concatenate Strings("Blank SN_", w437, w445) -> (w434:string)
                      n208 = Search 1D Array(1D array=w438, element=w434) -> (index of element=w436:i32)  [unwired: 1 in]
                      n209 = Less Than 0?(x=w436) -> (x < 0?=w435:bool)
                      n210 = Or(x=w435, y=w448) -> (x .or. y?=w447:bool)
                    }
                    n211 = Build Path(base path=w429, name or relative path=w427) -> (appended path=w430:path)
                  }
                }
                "Data Path" <- w393
                n212 = Empty String/Path?(string/path=w393) -> (empty?=w392:bool)
                n213 = case shown="False" w392 {
                  tunnel: w396 -> [w403 w407]
                  tunnel: [w403 w406] -> w395
                  frame True {
                    # "Cancelled"
                    n214 = local write "pb.RunSweeps"(FALSE ("pb.RunSweeps")) -> ()
                  }
                  frame False {
                    # "Continue"
                    n215 = Insert Into Array(array=w407, index=0, new element="Start Sweeps" ("new element/subarray")) -> (w406:string[])
                  }
                }
                n216 = Bundle By Name(cluster=w398, "Data Path"=w393) -> (w397:T12)
              }
            }
          }
          event "Bias Resistance", "Sweep Start Height", "Sweep End Height", "Sweep Time (s)", "Number of Sweeps", "Sweep PS Cmd": Value Change {
            n217 = event-data() -> ()  [unwired: 1 in, 6 out]
            n218 = Unbundle By Name("Test Header") -> ("Part Serial Number:"=w468:string, "Data Storage Folder:"=w453:path)
            n219 = call <vilib>:"Check if File or Folder Exists.vi"("path"=w453) -> ("error out"=w456:errorcluster, "file or folder exists?"=w455:bool, "dup path"=w454:path)  [unwired: 8 in]
            n220 = case shown="False" w455 {
              tunnel: w454 -> [w477 w480]
              tunnel: w456 -> [w476 _]
              tunnel: [w473 w480] -> w452
              frame False {
                # "DNE - Create"
                n221 = Create Folder(path (use dialog)=w477, error in=w476) -> (created path=w474:path, error out=w475:errorcluster)  [unwired: 1 in, 1 out]
                n222 = case shown="Error" w475 {
                  tunnel: w474 -> [w478 _]
                  tunnel: [w478 path "" ("created path")] -> w473
                  frame No Error {
                  }
                  frame Error {
                  }
                }
              }
              frame True {
                # "Exists - Continue"
              }
            }
            n223 = call "Remove Invalid File Characters.vi"("String In"=w468) -> ("String Out"=w464:string)  [unwired: 10 in]
            n224 = Bundle By Name(cluster=w467, "Test Params.Test Header"="Test Header", "Test Params.Test Header.Part Serial Number:"=w464, "Test Params.Test Header.Data Storage Folder:"=w452, "Test Params.Test Style"="Test Style", "Test Params.Bias Resistance"="Bias Resistance", "Test Params.Graph Parameters"="Graph Parameters", "Test Params.Test Parameters.Sweep Start Height"="Sweep Start Height", "Test Params.Test Parameters.Sweep End Height"="Sweep End Height", "Test Params.Test Parameters.Sweep Time (s)"="Sweep Time (s)", "Test Params.Test Parameters.Number of Sweeps"="Number of Sweeps", "Test Params.Test Parameters.Sweep PS Cmd"="Sweep PS Cmd") -> (w466:T12)
            n225 = Insert Into Array(array=w472, index=0, new element=string[] ["Update Controls", "Save Test Config", "Sweep Params to RT", "Sweep Enabler"]) -> (w471:string[])
          }
          event "pb.Open Test Config": Value Change {
            n226 = event-data() -> ()  [unwired: 1 in, 6 out]
            n227 = Unbundle By Name(w484) -> ("Config.Test Config Path"=w486:path)
            n228 = call "File Dialog"("start path"=w486) -> ("selected path"=w482:path, "cancelled"=w485:bool, "error out"=w481:errorcluster)  [unwired: 11 in, 1 out]
            n229 = call <vilib>:"Clear Errors.vi"("error in (no error)"=w481) -> ()  [unwired: 5 in, 2 out]
            n230 = case shown="False" w485 {
              tunnel: w488 -> [w495 w496]
              tunnel: [w494 w496] -> w487
              tunnel: w484 -> [w491 w497]
              tunnel: [w490 w497] -> w483
              tunnel: w482 -> [w489 _]
              frame False {
                n231 = Bundle By Name(cluster=w491, "Config.Test Config Path"=w489) -> (w490:T12)
                n232 = Insert Into Array(array=w495, index=0, new element=string[] ["Open Test Config", "Height Offset", "Update Controls", "Sweep Params to RT", "Write Controls", "Sweep Enabler"]) -> (w494:string[])
              }
              frame True {
              }
            }
          }
          event "pb.Copy Test Config": Value Change {
            n233 = event-data() -> ()  [unwired: 1 in, 1 out]
            n234 = Insert Into Array(array=w499, index=0, new element=string[] ["Copy Test Config"]) -> (w498:string[])
          }
          event "pb.Re-Run Graph": Value Change {
            n235 = event-data() -> ()  [unwired: 1 in, 1 out]
            n236 = Insert Into Array(array=w504, index=0, new element=string[] ["Finalize Sweeps 2"]) -> (w503:string[])
          }
          event "pb.Graph by File": Value Change {
            n237 = event-data() -> ()  [unwired: 1 in, 1 out]
            n238 = call "File Dialog3"() -> ("selected path"=w513:path, "cancelled"=w510:bool, "error out"=w509:errorcluster)  [unwired: 12 in, 1 out]
            n239 = Or(x=w510, y=w509) -> (x .or. y?=w508:bool)
            n240 = case shown="False" w508 {
              tunnel: w515 -> [w525 w528]
              tunnel: [w524 w528] -> w514
              tunnel: w513 -> [w518 _]
              tunnel: w512 -> [w520 w529]
              tunnel: [w519 w529] -> w511
              frame False {
                n241 = call-poly <vilib>:"Read Delimited Spreadsheet.vi"("file path (dialog if empty)"=w518, "delimiter (\\t)"="," ("delimiter (\\t)")) -> ("all rows"=w523:dbl[][])  [unwired: 8 in, 5 out]
                n242 = Delete From Array(array=w523, length=10, index (row)=0) -> (array with subset deleted=w517:dbl[][])  [unwired: 1 in, 1 out]
                n243 = Bundle By Name(cluster=w520, "Data Path"=w518, "Graph Data"=w517) -> (w519:T12)
                n244 = Insert Into Array(array=w525, index=0, new element=string[] ["Finalize Sweeps 2"]) -> (w524:string[])
              }
              frame True {
              }
            }
          }
        }
      }
      frame "Init" {
        w531 = T20."Disabled and Grayed Out" ("Disabled")
        w530 = FALSE ("pb.graph control")
        w551 = 0.0 ("Servo Control")
        n245 = flat-sequence {
          tunnel: [w556] -> w548
          tunnel: w547 -> [w556]
          tunnel: w548 -> [w558]
          frame #0 {
            n246 = call "Data (Global).vi"("Mode"=T17."Init") -> ()  [unwired: 11 in, 4 out]
          }
          frame #1 {
            n247 = Set Occurrence(w558) -> ()
          }
        }
        n248 = flat-sequence {
          tunnel: [w560] -> w550
          tunnel: w549 -> [w560]
          tunnel: w550 -> [w561]
          frame #0 {
            n249 = call "Graphing Data (global).vi"("Mode"=enum16{"Read", "Write", "Init", "Stop"}."Init") -> ()  [unwired: 12 in, 7 out]
          }
          frame #1 {
            n250 = Set Occurrence(w561) -> ()
          }
        }
        n251 = property class="App"() -> ("App.Kind"=w554:T16)  [unwired: 2 in, 2 out]
        n252 = local write "pb.graph control"(w530) -> ()
        n253 = local write "Connected?"(w530) -> ()
        n254 = local write "Connected? 2"(w530) -> ()
        n255 = local write "pb.RunSweeps"(w530) -> ()
        n256 = local write "pb.DO0"(w530) -> ()
        n257 = local write "pb.DO1"(w530) -> ()
        n258 = local write "pb.DO2"(w530) -> ()
        n259 = local write "pb.DO3"(w530) -> ()
        n260 = property on="led.DataWarning" class="Bool (strict)"("Visible"=FALSE) -> ()  [unwired: 2 in, 2 out]
        n261 = Equal?(x=w554, y=T16."Development System" ("Application:Kind")) -> (x = y?=w552:bool)
        n262 = call <vilib>:"Application Directory.vi"() -> ("Application Directory"=w544:path)
        n263 = property on="Screen" class="TabCtl (strict)"("Tabs Visible?"=w552) -> ()  [unwired: 2 in, 2 out]
        n264 = local write "led.DI 4"(w530) -> ()
        n265 = local write "led.DI 5"(w530) -> ()
        n266 = local write "led.DI 6"(w530) -> ()
        n267 = local write "led.DI 7"(w530) -> ()
        n268 = Build Path(base path=w544, name or relative path="Files\\Graphing Script") -> (appended path=w541:path)
        n269 = property on="pb.RunSweeps" class="Bool (strict)"("DisabledEnum"=w531) -> ()  [unwired: 2 in, 2 out]
        n270 = property on="pb.Re-Run Graph" class="Bool"("DisabledEnum"=w531) -> ()  [unwired: 2 in, 2 out]
        n271 = call "Create Python Graph.vi"("Python Script Directory"=w541, "Init (F)"=TRUE) -> ()  [unwired: 25 in, 1 out]
        n272 = local write "PS Command"(w551) -> ()
        n273 = local write "Spare Output"(w551) -> ()
        n274 = local write "Min Height"(w551) -> ()
        n275 = local write "Max Height"(w551) -> ()
        n276 = call <vilib>:"Application Directory.vi"() -> ("Application Directory"=w533:path)
        n277 = Build Path(base path=w533, name or relative path="Files\\Graphing Script") -> (appended path=w532:path)
        n278 = Bundle By Name(cluster=w536, "Graphing Script Dir"=w532) -> (w535:T12)
        n279 = Insert Into Array(array=w537, index=0, new element=string[] ["Open Test Config", "Height Offset", "Update Controls"]) -> (w538:string[])
        "led.DataWarning" <- TRUE ("led.DataWarning")
      }
      frame "Unused Items" {
      }
      frame "Load Config" {
        n280 = Unbundle By Name(w574) -> ("Config"=w572:T10)
        n281 = call <vilib>:"Application Directory.vi"() -> ("Application Directory"=w578:path)
        n282 = Build Path(base path=w578, name or relative path="Config.ini") -> (appended path=w567:path)
        n283 = call <vilib>:"Open Config Data.vi"("configuration file path"=w567) -> ("error out"=w575:errorcluster, "file created?"=w564:bool, "refnum"=w576:T25)  [unwired: 8 in]
        n284 = call <userlib>:"Read INI Cluster__ogtk.vi"("error in (no error)"=w575, "INI Fomatted Cluster Type"=w572, "refnum"=w576) -> ("error out"=w568:errorcluster, "INI Fomatted Cluster"=w571:variant, "dup refnum"=w569:T25)  [unwired: 4 in, 2 out]
        n285 = call <vilib>:"Close Config Data.vi"("error in (no error)"=w568, "refnum"=w569) -> ()  [unwired: 8 in, 2 out]
        n286 = Variant To Data(type=w572, Variant=w571) -> (data=w570:T10)  [unwired: 1 in, 1 out]
        n287 = case shown="True" w564 {
          tunnel: w566 -> [w579 w581]
          tunnel: [w579 w580] -> w565
          frame False {
          }
          frame True {
            n288 = Insert Into Array(array=w581, index=0, new element=string[] ["Save Config"]) -> (w580:string[])
          }
        }
        n289 = Bundle By Name(cluster=w574, "Config"=w570, "Config Path"=w567) -> (w573:T12)
      }
      frame "No IP" {
        n290 = Insert Into Array(array=w588, index=0, new element=string[] ["Unset Cursor Busy", "RIO Connection"]) -> (w585:string[])
        n291 = One Button Dialog(message="No IP address was found for the RIO. An IP address is necessary to connect.") -> ()  [unwired: 1 in, 1 out]
      }
      frame "Connect to RIO" {
        n292 = Unbundle By Name(w597) -> ("RIOTries"=w590:i32)
        n293 = case shown="0..4, Default" w590 {
          tunnel: [w604 string[] ["Unset Cursor Busy", "RIO Connection"]] -> w594
          tunnel: w590 -> [w603 _]
          tunnel: [w602 0] -> w591
          frame 0..4, Default {
            n294 = Increment(x=w603) -> (x+1=w602:i32)
            n295 = for {
              tunnel: string[] ["Connecting", "Connecting.", "Connecting..", "Connecting..."] -> [w605] mode=indexing
              n296 = property on="pb.connect" class="Bool (strict)"("BoolText.Text"=w605) -> ()  [unwired: 2 in, 2 out]
              n297 = Wait (ms)(milliseconds to wait=u32 200) -> ()  [unwired: 1 out]
            }
            n298 = And(x="Connected?", y="Connected? 2") -> (x .and. y?=w601:bool)
            n299 = case shown="True" w601 {
              tunnel: [string[] ["***MAIN***", "Connect to RIO"] string[] ["Connected", "Thaw Screen"]] -> w604
              frame False {
              }
              frame True {
              }
            }
          }
          frame 5 {
            n300 = flat-sequence {
              frame #0 {
                n301 = property on="pb.connect" class="Bool (strict)"("BoolText.Text"="FAILED" ("Boolean Text.Text")) -> ()  [unwired: 2 in, 2 out]
                n302 = Wait (ms)(milliseconds to wait=u32 500) -> ()  [unwired: 1 out]
              }
              frame #1 {
                n303 = property on="pb.connect" class="Bool (strict)"("BoolText.Text"="Connect\nto\nRIO" ("Boolean Text.Text")) -> ()  [unwired: 2 in, 2 out]
              }
            }
            n304 = local write "pb.connect"(FALSE ("pb.RetryRIO")) -> ()
          }
        }
        n305 = Bundle By Name(cluster=w597, "RIOTries"=w591) -> (w596:T12)
        n306 = Insert Into Array(array=w595, index=0, new element=w594) -> (w592:string[])
      }
      frame "Connected" {
        w639 = "Load Cal"
        n307 = Unbundle By Name(w620) -> ("Height Offset"=w615:dbl)
        n308 = local read "Sweep Start Height"() -> (w617:dbl)
        n309 = local read "Sweep End Height"() -> (w619:dbl)
        n310 = Flatten To String(anything=bool[] [FALSE, FALSE, FALSE, FALSE]) -> (data string=w661:string, error out=w651:errorcluster)  [unwired: 3 in, 1 out]
        n311 = Bundle("Digital Outputs", "data string"=w661) -> (w660:cluster{string, "data string":string})  [unwired: 1 in]
        n312 = Flatten To String(anything=w660, error in (no error)=w651) -> (data string=w659:string, error out=w650:errorcluster)  [unwired: 2 in, 1 out]
        n313 = call "PC Send Event.vi"("PC Send Command"=PCsend_RTrecv_CMD."Digital Outputs", "Mode"=Event_Mode."Set", "Flattened Data"=w659, "Error In"=w650) -> ("Error Out"=w649:errorcluster)  [unwired: 10 in, 1 out]
        n314 = Add(x=w615, y=w619) -> (x+y=w618:dbl)
        n315 = Add(x=w615, y=w617) -> (x+y=w616:dbl)
        n316 = local read "Number of Sweeps"() -> (w636:i32)
        n317 = local read "Sweep Time (s)"() -> (w638:dbl)
        n318 = Flatten To String(anything=dbl[] [0.0, 0.0, 0.0], error in (no error)=w649) -> (data string=w654:string, error out=w648:errorcluster)  [unwired: 2 in, 1 out]
        n319 = Bundle("Analog Outputs", "data string"=w654) -> (w653:cluster{string, "data string":string})  [unwired: 1 in]
        n320 = Flatten To String(anything=w653, error in (no error)=w648) -> (data string=w652:string, error out=w647:errorcluster)  [unwired: 2 in, 1 out]
        n321 = Multiply(x=w638, y=5000.0 ("x")) -> (x*y=w625:dbl)
        n322 = To Single Precision Float(number=w625) -> (single precision float=w629:sgl)
        n323 = To Single Precision Float(number=w618) -> (single precision float=w628:sgl)
        n324 = To Single Precision Float(number=w616) -> (single precision float=w627:sgl)
        n325 = To Single Precision Float(number=w636) -> (single precision float=w621:sgl)
        n326 = call "PC Send Event.vi"("PC Send Command"=PCsend_RTrecv_CMD."Analog Outputs", "Mode"=Event_Mode."Set", "Flattened Data"=w652, "Error In"=w647) -> ("Error Out"=w640:errorcluster)  [unwired: 10 in, 1 out]
        n327 = property on="Screen" class="TabCtl (strict)"("Value"=T15."Run Screen" ("Screen")) -> ()  [unwired: 2 in, 2 out]
        n328 = Insert Into Array(array=w668, index=0, new element=string[] ["Unset Cursor Busy"]) -> (w667:string[])
        n329 = Build Array(w629, w628, w627, w621) -> (w626:sgl[])
        n330 = Bundle(w639, w639) -> (w643:cluster{string, string})  [unwired: 1 in]
        n331 = Flatten To String(anything=w643, error in (no error)=w640) -> (data string=w644:string, error out=w645:errorcluster)  [unwired: 2 in, 1 out]
        n332 = call "PC Send Event.vi"("PC Send Command"=PCsend_RTrecv_CMD."Load Cal", "Mode"=Event_Mode."Set", "Flattened Data"=w644, "Error In"=w645) -> ("Error Out"=w624:errorcluster)  [unwired: 10 in, 1 out]
        n333 = Flatten To String(anything=w626, error in (no error)=w624) -> (data string=w632:string, error out=w623:errorcluster)  [unwired: 2 in, 1 out]
        n334 = Bundle("Sweep Parameters", "data string"=w632) -> (w631:cluster{string, "data string":string})  [unwired: 1 in]
        n335 = Flatten To String(anything=w631, error in (no error)=w623) -> (data string=w630:string, error out=w622:errorcluster)  [unwired: 2 in, 1 out]
        n336 = call "PC Send Event.vi"("PC Send Command"=PCsend_RTrecv_CMD."Sweep Parameters", "Mode"=Event_Mode."Set", "Flattened Data"=w630, "Error In"=w622) -> ()  [unwired: 10 in, 2 out]
      }
      frame "Open Test Config" {
        n337 = Unbundle By Name(w672) -> ("Test Params"=w674:T8, "Config.Test Config Path"=w671:path)
        n338 = call <vilib>:"Check if File or Folder Exists.vi"("path"=w671) -> ("file or folder exists?"=w670:bool)  [unwired: 8 in, 2 out]
        n339 = case shown="True" w670 {
          tunnel: w676 -> [w677 w689]
          tunnel: [w677 w688] -> w675
          tunnel: w674 -> [_ w687]
          tunnel: [w678 w686] -> w673
          tunnel: w672 -> [w678 w685]
          tunnel: w671 -> [_ w681]
          frame False {
          }
          frame True {
            n340 = Read from Binary File(5:w687, 11:w681) -> (2:w680:T8)  [unwired: 4 in, 3 out]
            n341 = Strip Path(path=w681) -> (name=w682:string)  [unwired: 1 out]
            "Test Config" <- w682
            n342 = Unbundle By Name(w680) -> ("Height Offset"=w679:dbl)
            n343 = Bundle By Name(cluster=w685, "Test Params"=w680, "Test Config"=w682, "Config.Test Config Path"=w681, "Height Offset"=w679) -> (w686:T12)
            n344 = Insert Into Array(array=w689, index=0, new element=string[] ["Save Config"]) -> (w688:string[])
          }
        }
      }
      frame "Copy Test Config" {
        n345 = Unbundle By Name(w691) -> ("Test Params"=w693:T8, "Config.Test Config Path"=w696:path)
        n346 = call "File Dialog2"("start path"=w696) -> ("selected path"=w694:path, "cancelled"=w695:bool, "error out"=w690:errorcluster)  [unwired: 11 in, 1 out]
        n347 = call <vilib>:"Clear Errors.vi"("error in (no error)"=w690) -> ()  [unwired: 5 in, 2 out]
        n348 = case shown="False" w695 {
          tunnel: w698 -> [w706 w708]
          tunnel: [w705 w708] -> w697
          tunnel: w694 -> [w699 _]
          tunnel: w693 -> [w701 _]
          tunnel: w691 -> [w703 w709]
          tunnel: [w702 w709] -> w692
          frame False {
            n349 = Write to Binary File(file (use dialog)=w699, data=w701) -> ()  [unwired: 4 in, 3 out]
            n350 = Strip Path(path=w699) -> (name=w700:string)  [unwired: 1 out]
            n351 = local write "Test Config"(w700) -> ()
            n352 = Bundle By Name(cluster=w703, "Config.Test Config Path"=w699, "Test Config"=w700) -> (w702:T12)
            n353 = Insert Into Array(array=w706, index=0, new element=string[] ["Save Config"]) -> (w705:string[])
          }
          frame True {
          }
        }
      }
      frame "Height Offset" {
        n354 = Unbundle By Name(w712) -> ("Test Params.Height Offset"=w710:dbl, "Height Offset"=w713:dbl, "Controls"=w718:dbl[])
        n355 = Index Array(array=w718) -> (element=w717:dbl)  [unwired: 1 in]
        n356 = Subtract(x=w710, y=w713) -> (x-y=w716:dbl)
        n357 = Subtract(x=w717, y=w716) -> (x-y=w715:dbl)
        n358 = Replace Array Subset(array=w718, new element=w715) -> (w714:dbl[])  [unwired: 1 in]
        n359 = local write "Cal Controls:"(w714) -> ()
        n360 = local write "Position Command"(w715) -> ()
        n361 = Bundle By Name(cluster=w712, "Height Offset"=w710, "Controls"=w714) -> (w711:T12)
        n362 = Insert Into Array(array=w722, index=0, new element=string[] []) -> (w721:string[])
      }
      frame "Save Test Config" {
        n363 = Unbundle By Name(w725) -> ("Height Offset"=w723:dbl)
        n364 = Bundle By Name(cluster=w725, "Test Params.Height Offset"=w723) -> (w724:T12)
        n365 = Unbundle By Name(w724) -> ("Config.Test Config Path"=w727:path, "Test Params"=w726:T8)
        n366 = Write to Binary File(file (use dialog)=w727, data=w726) -> ()  [unwired: 4 in, 3 out]
        n367 = Insert Into Array(array=w730, index=0, new element=string[] []) -> (w729:string[])
      }
      frame "Sweep Params to RT" {
        # "Sweep Time (s) X 10kHz X 0.5 FPGA time is one-directional"
        n368 = Unbundle By Name(w737) -> ("Test Params.Height Offset"=w732:dbl, "Test Params.Test Parameters.Sweep Time (s)"=w736:dbl, "Test Params.Test Parameters.Sweep Start Height"=w735:dbl, "Test Params.Test Parameters.Sweep End Height"=w734:dbl, "Test Params.Test Parameters.Number of Sweeps"=w733:i32)
        n369 = Add(x=w732, y=w734) -> (x+y=w744:dbl)
        n370 = Add(x=w732, y=w735) -> (x+y=w743:dbl)
        n371 = Multiply(x=w736, y=5000.0 ("x")) -> (x*y=w748:dbl)
        n372 = To Single Precision Float(number=w748) -> (single precision float=w751:sgl)
        n373 = To Single Precision Float(number=w744) -> (single precision float=w750:sgl)
        n374 = To Single Precision Float(number=w743) -> (single precision float=w749:sgl)
        n375 = To Single Precision Float(number=w733) -> (single precision float=w745:sgl)
        n376 = Build Array(w751, w750, w749, w745) -> (w742:sgl[])
        n377 = Flatten To String(anything=w742) -> (data string=w754:string, error out=w747:errorcluster)  [unwired: 3 in, 1 out]
        n378 = Bundle("Sweep Parameters", "data string"=w754) -> (w753:cluster{string, "data string":string})  [unwired: 1 in]
        n379 = Flatten To String(anything=w753, error in (no error)=w747) -> (data string=w752:string, error out=w746:errorcluster)  [unwired: 2 in, 1 out]
        n380 = call "PC Send Event.vi"("PC Send Command"=PCsend_RTrecv_CMD."Sweep Parameters", "Mode"=Event_Mode."Set", "Flattened Data"=w752, "Error In"=w746) -> ()  [unwired: 10 in, 2 out]
        n381 = Insert Into Array(array=w757, index=0, new element=string[] []) -> (w756:string[])
      }
      frame "Update Controls" {
        n382 = Unbundle By Name(w768) -> ("Test Params.Test Header"=w767:T7, "Test Params.Test Style"=w766:T2, "Test Params.Bias Resistance"=w765:dbl, "Test Params.Graph Parameters"=w764:T3, "Test Params.Test Parameters.Sweep Start Height"=w763:dbl, "Test Params.Test Parameters.Sweep End Height"=w762:dbl, "Test Params.Test Parameters.Sweep Time (s)"=w761:dbl, "Test Params.Test Parameters.Sweep PS Cmd"=w760:dbl, "Test Params.Test Parameters.Number of Sweeps"=w759:i32)
        n383 = local write "Test Header"(w767) -> ()
        n384 = local write "Test Style"(w766) -> ()
        n385 = local write "Bias Resistance"(w765) -> ()
        n386 = local write "Graph Parameters"(w764) -> ()
        n387 = local write "Sweep Start Height"(w763) -> ()
        n388 = local write "Sweep End Height"(w762) -> ()
        n389 = local write "Sweep Time (s)"(w761) -> ()
        n390 = local write "Sweep PS Cmd"(w760) -> ()
        n391 = local write "Number of Sweeps"(w759) -> ()
        n392 = Insert Into Array(array=w771, index=0, new element=string[] []) -> (w770:string[])
      }
      frame "Read Data" {
        # "Swithed from first to last\nwith storing more data"
        # "Formerly determined Save Sweeps"
        # "Had used an AND on Sweeps like on graph, but that prevents finding the last sweep"
        # "Check Sweeps case runs 10x faster\nSo it finds the sweep is done,\nstill save once more to get final data"
        n393 = Unbundle By Name(w831) -> ("Height Offset"=w817:dbl, "Graph Active"=w829:bool, "SweepsRunning"=w777:bool, "Test Params.Bias Resistance"=w807:dbl)
        n394 = call "Data (Global).vi"("Mode"=T17."Read Data") -> ("Data Out"=w819:dbl[][], "New Data"=w788:bool, "OverwriteErr#"=w781:i32, "StreamErr#"=w780:i32)  [unwired: 11 in]
        n395 = call "Evaluate Data Errors.vi"("Overwrite Error"=w781, "Stream Error"=w780, "Sweeps Running"=w777) -> ("Data Error"=w779:bool)  [unwired: 12 in]
        n396 = property on="led.DataWarning" class="Bool (strict)"("Visible"=w779) -> ()  [unwired: 2 in, 2 out]
        n397 = feedback-in #2(w777) -> ()
        n398 = feedback #2(w777) -> (w778:bool)
        n399 = feedback #3(0 ("t")) -> (w800:i32)
        n400 = Select(t=11, s=w777, f=w800) -> (s? t:f=w797:i32)
        n401 = Decrement(x=w797) -> (x-1=w802:i32)
        n402 = Less Than 0?(x=w802) -> (x < 0?=w803:bool)
        n403 = Or(x=w778, y=w777) -> ()  [unwired: 1 out]
        n404 = Less?(x=w778, y=w777) -> (x < y?=w776:bool)
        n405 = Equal?(x=1, y=w797) -> (x = y?=w795:bool)
        n406 = Select(t=0, s=w803, f=w802) -> (s? t:f=w798:i32)
        n407 = feedback-in #3(w798) -> ()
        n408 = And(x=w788, y=w829) -> (x .and. y?=w827:bool)
        n409 = Transpose 2D Array(2D array=w819) -> (transposed array=w787:dbl[][])
        n410 = Greater Than 0?(x=w798) -> (x > 0?=w775:bool)
        n411 = case shown="True" w827 {
          tunnel: w828 -> [w842 w844]
          tunnel: [w842 w843] -> w824
          frame False {
          }
          frame True {
            n412 = Insert Into Array(array=w844, index=0, new element=string[] ["Graph"]) -> (w843:string[])
          }
        }
        n413 = Index Array(array=w787, index (col)=3 ("index (row)")) -> (element=w823:dbl[])  [unwired: 1 in]
        n414 = Array Size(array=w787) -> (size(s)=w786:i32[])
        n415 = Select(t=FALSE, s=w776, f=w775) -> (s? t:f=w774:bool)
        n416 = Subtract(x=w823, y=w817) -> (x-y=w822:dbl[])
        n417 = Index Array(array=w786, index=0) -> (element=w784:i32)
        n418 = Insert Into Array(array=w787, index (col)=4 ("index (row)"), new element=w822) -> (w818:dbl[][])  [unwired: 1 in]
        n419 = Decrement(x=w784) -> (x-1=w783:i32)
        n420 = Index Array(array=w818, index (row)=w783) -> (element=w820:dbl[])  [unwired: 1 in]
        "Cal Readings:" <- w820
        n421 = Not A Number/Path/Refnum?(number/path/refnum=w807) -> (NaN/Path/Refnum?=w806:bool)
        n422 = case shown="True" w774 {
          tunnel: w824 -> [w837 w839]
          tunnel: [w837 w838] -> w794
          frame False {
          }
          frame True {
            n423 = Insert Into Array(array=w839, index=0, new element=string[] ["Save Sweeps"]) -> (w838:string[])
          }
        }
        n424 = Index Array(array=w820) -> (element #1=w814:dbl, element #2=w813:dbl, element #3=→"Spare":dbl, element #4=→"Abs. Height":dbl, element #5=→"Relative Height":dbl)  [unwired: 5 in]
        "PS Volt" <- w814
        "LS Volt" <- w813
        n425 = Subtract(x=w814, y=w813) -> (x-y=w808:dbl)
        n426 = Divide(x=w813, y=w808) -> (x/y=w812:dbl)
        n427 = Multiply(x=w812, y=w807) -> (x*y=w811:dbl)
        n428 = Equal To 0?(x=w808) -> (x = 0?=w805:bool)
        n429 = Or(x=w806, y=w805) -> (x .or. y?=w804:bool)
        n430 = Select(t=nan, s=w804, f=w811) -> (s? t:f=→"Resistance":dbl)
        n431 = Compound Arithmetic op=AND(w795, invert w774) -> (w793:bool)
        n432 = Get Date/Time In Seconds() -> (seconds since 1Jan1904=w790:timestamp)
        n433 = To Double Precision Float(number=w790) -> (double precision float=w789:dbl)
        n434 = case shown="True" w793 {
          tunnel: w794 -> [w832 w834]
          tunnel: [w832 w833] -> w792
          frame False {
          }
          frame True {
            n435 = Insert Into Array(array=w834, index=0, new element=string[] ["Finalize Sweeps"]) -> (w833:string[])
          }
        }
        n436 = Bundle By Name(cluster=w831, "New Data"=w788, "Data"=w818, "Data_Current"=w820, "Data Clock"=w789) -> (w830:T12)
      }
      frame "Write Controls" {
        w861 = 3 ("length")
        w862 = 4 ("index")
        # "Position Command calibration now handled on FPGA"
        n437 = local read "Screen"() -> (w850:T1)
        n438 = Equal?(x=w850, y=T15."Calibration" ("Screen")) -> (x = y?=w849:bool)
        n439 = case shown="False" w849 {
          tunnel: w865 -> [w871 w876]
          tunnel: [w870 w873] -> w864
          tunnel: [w869 w874] -> w863
          tunnel: [w868 w875] -> w860
          tunnel: [w867 w872] -> w847
          frame False {
            n440 = Unbundle By Name(w871) -> ("Height Offset"=w867:dbl, "Controls"=w868:dbl[], "Slope Values"=w870:dbl[], "Offset Values"=w869:dbl[])
          }
          frame True {
            n441 = local read "Offset Values:"() -> (w874:dbl[])
            n442 = Unbundle By Name(w876) -> ("Height Offset"=w872:dbl, "Controls"=w875:dbl[])
            n443 = local read "Slope Values:"() -> (w873:dbl[])
          }
        }
        n444 = Array Subset(array=w864, index=w862, length=w861) -> (w859:dbl[])
        n445 = Array Subset(array=w863, index=w862, length=w861) -> (w858:dbl[])
        n446 = for {
          tunnel: w860 -> [w883] mode=indexing
          tunnel: w859 -> [w882] mode=indexing
          tunnel: w858 -> [w881] mode=indexing
          tunnel: [w880] -> w851 mode=indexing
          tunnel: w847 -> [w877]
          i -> [w879]
          n447 = Equal To 0?(x=w879) -> (x = 0?=w878:bool)
          n448 = case shown="True" w878 {
            tunnel: w883 -> [w886 w891]
            tunnel: w882 -> [_ w890]
            tunnel: w881 -> [_ w888]
            tunnel: [w884 w887] -> w880
            tunnel: w877 -> [w885 _]
            frame True {
              n449 = Add(x=w886, y=w885) -> (x+y=w884:dbl)
            }
            frame False {
              n450 = Multiply(x=w891, y=w890) -> (x*y=w889:dbl)
              n451 = Add(x=w889, y=w888) -> (x+y=w887:dbl)
            }
          }
        }
        n452 = Flatten To String(anything=w851) -> (data string=w854:string)  [unwired: 3 in, 2 out]
        n453 = Bundle("Analog Outputs", "data string"=w854) -> (w853:cluster{string, "data string":string})  [unwired: 1 in]
        n454 = Flatten To String(anything=w853) -> (data string=w852:string)  [unwired: 3 in, 2 out]
        n455 = call "PC Send Event.vi"("PC Send Command"=PCsend_RTrecv_CMD."Analog Outputs", "Mode"=Event_Mode."Set", "Flattened Data"=w852) -> ()  [unwired: 11 in, 2 out]
      }
      frame "Graph" {
        n456 = Unbundle By Name(w893) -> ("Data"=→"Chart":dbl[][])
      }
      frame "Save Cal" {
        n457 = Unbundle By Name(w899) -> ("Slope Values"=w898:dbl[], "Gauge#"=w896:i32, "CalDueDate"=w895:string, "Offset Values"=w897:dbl[])
        n458 = disable-structure shown="Disabled" {
          disable-tunnel: w898 -> [w913 _]
          disable-tunnel: w897 -> [w912 _]
          disable-tunnel: w896 -> [w911 _]
          disable-tunnel: w895 -> [w910 _]
          frame Disabled {
            n459 = Bundle By Name(cluster=T18 {"Slope"=[], "Offset"=[], "Gauge#"=0, "CalDueDate"=""}, "Slope"=w913, "Offset"=w912, "Gauge#"=w911, "CalDueDate"=w910) -> (w901:T18)
            n460 = Flatten To String(anything=w901) -> (data string=w906:string, error out=w903:errorcluster)  [unwired: 3 in, 1 out]
            n461 = Bundle("Cal2RT", "data string"=w906) -> (w905:cluster{string, "data string":string})  [unwired: 1 in]
            n462 = Flatten To String(anything=w905, error in (no error)=w903) -> (data string=w904:string, error out=w902:errorcluster)  [unwired: 2 in, 1 out]
            n463 = call "PC Send Event.vi"("PC Send Command"=PCsend_RTrecv_CMD."Cal2RT", "Mode"=Event_Mode."Set", "Flattened Data"=w904, "Error In"=w902) -> ()  [unwired: 10 in, 2 out]
          }
          frame Enabled {
          }
        }
        n464 = disable-structure shown="Disabled" {
          disable-tunnel: w898 -> [w918 _]
          disable-tunnel: w897 -> [w917 _]
          disable-tunnel: w896 -> [w916 _]
          disable-tunnel: w895 -> [w915 _]
          frame Disabled {
            w920 = ""
            n465 = Number To Decimal String(number=w916) -> (decimal integer string=w919:string)  [unwired: 1 in]
            n466 = Number To Fractional String(number=w918) -> (F-format string=w924:string[])  [unwired: 3 in]
            n467 = Number To Fractional String(number=w917) -> (F-format string=w922:string[])  [unwired: 3 in]
            n468 = Build Array (concatenate)(w924, w919, w915) -> (w923:string[])
            n469 = Build Array (concatenate)(w922, w920, w920) -> (w921:string[])
            n470 = Replace Array Subset(array=string[][] [["Power Supply Voltage", "Level Sender Voltage", "AI-3 Spare", "Height Gauge", "Servo Motor Control", "Spare Analog Output 1", "Spare Analog Output 2", "Gauge Number", "CalDueDate"], ["", "", "", "", "", "", "", "", ""], ["", "", "", "", "", "", "", "", ""]], new element=w923, index (row)=1) -> (w932:string[][])  [unwired: 1 in]
            n471 = Replace Array Subset(array=w932, new element=w921, index (row)=2) -> (w931:string[][])  [unwired: 1 in]
            n472 = Insert Into Array(array=w931, index (col)=0 ("disabled index (col)"), new element=string[] ["Channel Name", "Slope", "Offset"]) -> (w926:string[][])  [unwired: 1 in]
            n473 = Array To Spreadsheet String(delimiter (Tab)=",", array=w926, 3:"%s" ("format string")) -> (spreadsheet string=w937:string)
            n474 = Open/Create/Replace File(file path (use dialog)=path "u:/Internal.cal", operation (0:open)=T19."replace or create") -> (refnum out=w934:refnum<file>, error out=w933:errorcluster)  [unwired: 4 in, 1 out]
            n475 = Write to Text File(file (use dialog)=w934, text=w937, error in=w933) -> (refnum out=w941:refnum<file>, error out=w942:errorcluster)  [unwired: 1 in, 1 out]
            n476 = Close File(refnum=w941, error in=w942) -> (error out=w940:errorcluster)  [unwired: 1 out]
            n477 = call <vilib>:"Clear Errors.vi"("error in (no error)"=w940) -> ()  [unwired: 5 in, 2 out]
          }
          frame Enabled {
          }
        }
      }
      frame "Sweep Enabler" {
        n478 = Unbundle By Name(w970) -> ("Test Params.Graph Parameters.Height Min"=w963:i32, "Test Params.Graph Parameters.Height Max"=w952:i32, "Test Params.Graph Parameters.Height Interval"=w951:i32, "Test Params.Graph Parameters.Res Max"=w950:i32, "Test Params.Graph Parameters.Res Interval"=w949:i32, "Test Params.Graph Parameters.Time Max"=w948:i32, "Test Params.Graph Parameters.Time Interval"=w947:i32, "Test Params.Test Parameters.Sweep Time (s)"=w969:dbl, "Test Params.Test Parameters.Sweep End Height"=w968:dbl, "Test Params.Test Parameters.Sweep Start Height"=w967:dbl, "Test Params.Test Parameters.Number of Sweeps"=w966:i32, "Test Params.Test Header.CA Number:"=w962:string, "Test Params.Test Header.Part Model:"=w961:string, "Test Params.Test Header.Part Serial Number:"=w960:string, "Test Params.Test Header.Technician Name:"=w959:string, "Test Params.Test Header.Test Fluid:"=w958:string, "Test Params.Test Header.Hours Description:"=w957:string, "Test Params.Test Header.Data Storage Folder:"=w954:path)
        n479 = Path To String(path=w954) -> (string=w953:string)
        n480 = Build Array(w952, w951, w950, w949, w948, w947) -> (w946:i32[])
        n481 = Build Array(w962, w961, w960, w959, w958, w957, w953) -> (w956:string[])
        n482 = Empty String/Path?(string/path=w956) -> (empty?=w965:bool[])
        n483 = Not Equal?(x=w963, y=w952) -> (x != y?=w943:bool)
        n484 = Not Equal To 0?(x=w946) -> (x != 0?=w945:bool[])
        n485 = Not Equal To 0?(x=w969) -> (x != 0?=w978:bool)
        n486 = Not Equal To 0?(x=w968) -> (x != 0?=w977:bool)
        n487 = Not Equal?(x=w968, y=w967) -> (x != y?=w971:bool)
        n488 = Not Equal To 0?(x=w966) -> (x != 0?=w972:bool)
        n489 = Not(x=w965) -> (.not. x?=w964:bool[])
        n490 = And Array Elements(Boolean array=w945) -> (logical AND=w944:bool)
        n491 = And Array Elements(Boolean array=w964) -> (logical AND=w955:bool)
        n492 = Compound Arithmetic op=AND(w943, w944, w978, w977, w971, w972, w955) -> (w976:bool)
        n493 = Select(t=T20."Enabled" ("Disabled"), s=w976, f=T20."Disabled and Grayed Out" ("Disabled")) -> (s? t:f=w973:T20)
        n494 = property on="pb.RunSweeps" class="Bool (strict)"("DisabledEnum"=w973) -> ()  [unwired: 2 in, 2 out]
      }
      frame "Start Sweeps" {
        w988 = string[][] [["Test Style:", "CA Number:", "Part Serial Number:", "Part Model:", "Technician Name:"], ["", "", "", "", ""], ["Start Time:", "Sampling Interval:", "Total Time:", "Start Position:", "End Position:"], ["", "", "", "", ""], ["Bias Resistance:", "Height Offset (mm):", "Test Fluid:", "Gauge Number:", "Cal Due Date:"], ["", "", "", "", ""], ["Hours Description:", "", "", "", ""], ["", "", "", "", ""], ["", "", "", "", ""], ["Time Elapsed (s):", "Height (mm):", "LS Voltage (V):", "Applied Voltage (V):", "LS Resistance (ohms):"]]  # Header Template
        w996 = 0.0 ("MaxResistance")
        # "Start Sweeps"
        n495 = Unbundle By Name(w1043) -> ("Test Params.Test Header.Hours Description:"=w995:string, "Test Params.Bias Resistance"=w999:dbl, "Test Params.Test Header.Test Fluid:"=w985:string, "Data Path"=w1034:path, "Height Offset"=w1033:dbl, "Gauge#"=w1022:i32, "CalDueDate"=w1020:string, "Test Params.Test Parameters.Number of Sweeps"=w1015:i32, "Test Params.Test Parameters.Sweep Time (s)"=w1014:dbl, "Test Params.Test Parameters.Sweep Start Height"=w1018:dbl, "Test Params.Test Parameters.Sweep End Height"=w1019:dbl, "Test Params.Test Style"=w987:T2, "Test Params.Test Header.CA Number:"=w984:string, "Test Params.Test Header.Part Serial Number:"=w997:string, "Test Params.Test Header.Part Model:"=w983:string, "Test Params.Test Header.Technician Name:"=w982:string, "Controls"=w1002:dbl[], "Test Params.Test Parameters.Sweep PS Cmd"=w981:dbl)
        n496 = Get Date/Time In Seconds() -> (seconds since 1Jan1904=w1029:timestamp)
        n497 = Replace Array Subset(array=string[] ["", "", "", "", ""], new element=w995, index=0) -> (w990:string[])
        n498 = Format Date/Time String(time format string (%c)="%m/%d/%Y %I:%M:%S %p ", seconds (now)=w1029) -> (date/time string=w1024:string)  [unwired: 1 in]
        n499 = Multiply(x=w1015, y=w1014) -> (x*y=w1013:dbl)
        n500 = Format Into String(w987) -> (resulting string=w986:string)  [unwired: 3 in, 1 out]
        n501 = Number To Fractional String(number=w1013) -> (F-format string=w1012:string)  [unwired: 3 in]
        n502 = Number To Fractional String(number=w1018) -> (F-format string=w1016:string)  [unwired: 3 in]
        n503 = Number To Fractional String(number=w1019) -> (F-format string=w1017:string)  [unwired: 3 in]
        n504 = Number To Fractional String(number=w999) -> (F-format string=w1027:string)  [unwired: 3 in]
        n505 = Number To Fractional String(number=w1033) -> (F-format string=w1026:string)  [unwired: 3 in]
        n506 = Number To Decimal String(number=w1022) -> (decimal integer string=w1021:string)  [unwired: 1 in]
        n507 = Build Array(w1024, "0.0005s" ("time format string (%c)"), w1012, w1016, w1017) -> (w1008:string[])
        n508 = Build Array(w986, w984, w997, w983, w982) -> (w1009:string[])
        n509 = Build Array(w1027, w1026, w985, w1021, w1020) -> (w991:string[])
        n510 = Replace Array Subset(array=w1002, new element=w981, index=1) -> (w1000:dbl[])
        n511 = Insert Into Array(array=w1045, index=0, new element=string[] ["Write Controls", "Handle Disables", "Init FPGA Sweeps"]) -> (w1044:string[])
        n512 = local write "Cal Controls:"(w1000) -> ()
        n513 = local write "PS Command"(w981) -> ()
        n514 = Open/Create/Replace File(file path (use dialog)=w1034, operation (0:open)=T19."replace or create") -> (refnum out=w1036:refnum<file>, error out=w1035:errorcluster)  [unwired: 4 in, 1 out]
        n515 = Replace Array Subset(array=w988, new element=w990, index (row)=7) -> (w992:string[][])  [unwired: 1 in]
        n516 = Replace Array Subset(array=w992, new element=w991, index (row)=5) -> (w1011:string[][])  [unwired: 1 in]
        n517 = Replace Array Subset(array=w1011, new element=w1008, index (row)=3) -> (w1010:string[][])  [unwired: 1 in]
        n518 = Replace Array Subset(array=w1010, new element=w1009, index (row)=1) -> (w1004:string[][])  [unwired: 1 in]
        n519 = Array To Spreadsheet String(delimiter (Tab)=",", array=w1004, 3:"%s" ("format string")) -> (spreadsheet string=w1031:string)
        n520 = Write to Text File(file (use dialog)=w1036, text=w1031, error in=w1035) -> (refnum out=w1039:refnum<file>, error out=w1040:errorcluster)  [unwired: 1 in, 1 out]
        n521 = Close File(refnum=w1039, error in=w1040) -> (error out=w1038:errorcluster)  [unwired: 1 out]
        n522 = call <vilib>:"Clear Errors.vi"("error in (no error)"=w1038) -> ()  [unwired: 5 in, 2 out]
        n523 = local write "Max Height"(w996) -> ()
        n524 = Bundle By Name(cluster=w1043, "Graph Data"=dbl[][] [], "FinalizeSweeps"=FALSE, "Data Index"=0, "Controls"=w1000, "MaxResistance"=w996, "Min Height"=w996, "Max Height"=w996) -> (w1042:T12)
        n525 = local write "Min Height"(w996) -> ()
      }
      frame "Init FPGA Sweeps" {
        n526 = flat-sequence {
          tunnel: w1050 -> [w1052]
          tunnel: [w1052] -> w1049
          tunnel: [w1062] -> w1048
          tunnel: w1049 -> [w1063]
          frame #0 {
            # "Does not count towards\nsave time"
            # "To make sure power is on and\nresistance is right"
            n527 = Wait (ms)(milliseconds to wait=u32 250) -> ()  [unwired: 1 out]
          }
          frame #1 {
            w1058 = 1000.0  # Data Rate
            # "Changed Data rate from 2k to 1k"
            # "End buffer minus zero-based"
            n528 = Unbundle By Name(w1063) -> ("Graph Active"=w1064:bool, "Test Params.Test Parameters.Sweep Time (s)"=w1061:dbl, "Test Params.Test Parameters.Number of Sweeps"=w1060:i32)
            n529 = Multiply(x=w1061, y=w1060) -> (x*y=w1059:dbl)
            n530 = Multiply(x=w1059, y=w1058) -> (x*y=w1056:dbl)
            n531 = Add(x=w1056, y=549.0) -> (x+y=w1054:dbl)
            n532 = case shown="False" w1064 {
              tunnel: w1063 -> [w1078 w1083]
              tunnel: [w1077 w1083] -> w1062
              tunnel: w1054 -> [w1074 w1082]
              tunnel: [w1072 w1079] -> w1057
              frame False {
                w1076 = TRUE ("Graph Active")
                # "Not graphing - clear, format, and start"
                n533 = Bundle By Name(cluster=w1078, "Graph Active"=w1076) -> (w1077:T12)
                n534 = local write "pb.graph control"(w1076) -> ()
                n535 = property on="Chart" class="WFChart (strict)"("History Data"=dbl[][] [], "XScale.Minimum"=0.0 ("X Scale.Range:Minimum"), "XScale.Maximum"=w1074) -> (error out=w1072:errorcluster)  [unwired: 2 in, 1 out]
              }
              frame True {
                # "Already graphing - nothing changes"
                n536 = property on="Chart" class="WFChart (strict)"() -> ("XScale.Minimum"=w1081:dbl)  [unwired: 2 in, 2 out]
                n537 = Add(x=w1081, y=w1082) -> (x+y=w1080:dbl)
                n538 = property on="Chart" class="WFChart (strict)"("XScale.Maximum"=w1080) -> (error out=w1079:errorcluster)  [unwired: 2 in, 1 out]
              }
            }
            n539 = Flatten To String(anything=TRUE, error in (no error)=w1057) -> (data string=w1068:string)  [unwired: 2 in, 2 out]
            n540 = Bundle("Start Sweep", "data string"=w1068) -> (w1067:cluster{string, "data string":string})  [unwired: 1 in]
            n541 = Flatten To String(anything=w1067) -> (data string=w1066:string)  [unwired: 3 in, 2 out]
            n542 = call "PC Send Event.vi"("PC Send Command"=PCsend_RTrecv_CMD."Start Sweep", "Mode"=Event_Mode."Set", "Flattened Data"=w1066) -> ()  [unwired: 11 in, 2 out]
          }
        }
        n543 = Bundle By Name(cluster=w1048, "SweepsRunning"=TRUE) -> (w1047:T12)
      }
      frame "Check Sweeps" {
        n544 = disable-structure shown="Disabled" {
          disable-tunnel: w1087 -> [w1110 w1190]
          disable-tunnel: [w1109 w1190] -> w1086
          disable-tunnel: w1085 -> [w1104 w1189]
          disable-tunnel: [w1103 w1189] -> w1084
          frame Disabled {
            n545 = Unbundle By Name(w1110) -> ("Controls"=w1114:dbl[], "SweepsForward"=w1094:bool, "Data_Current"=w1112:dbl[], "Sweep Start Ht"=w1093:dbl, "Sweep End Ht"=w1092:dbl, "Sweep Time"=w1095:dbl, "SweepsSwept"=w1107:i32, "# of Sweeps"=w1106:i32, "Waveform"=w1091:dbl[], "Current Point"=w1090:i32, "Wave.pts"=w1089:i32)
            n546 = disable-structure shown="Enabled" {
              disable-tunnel: w1112 -> [w1127 _]
              disable-tunnel: [w1124 w1176] -> w1111
              disable-tunnel: [w1123 TRUE] -> w1108
              disable-tunnel: w1107 -> [w1122 w1174]
              disable-tunnel: w1106 -> [w1121 w1173]
              disable-tunnel: [w1120 w1172] -> w1105
              disable-tunnel: [w1119 w1171] -> w1096
              disable-tunnel: w1095 -> [w1118 _]
              disable-tunnel: w1094 -> [w1117 _]
              disable-tunnel: w1093 -> [w1116 _]
              disable-tunnel: w1092 -> [w1115 _]
              disable-tunnel: w1091 -> [_ w1177]
              disable-tunnel: w1089 -> [_ w1181]
              disable-tunnel: w1090 -> [_ w1182]
              disable-tunnel: [_ w1170] -> w1088
              frame Disabled {
                n547 = Index Array(array=w1127, index=4) -> (element=w1125:dbl)
                n548 = case shown="False" w1117 {
                  tunnel: w1125 -> [w1129 w1164]
                  tunnel: w1115 -> [_ w1163]
                  tunnel: w1118 -> [w1133 w1161]
                  tunnel: [w1132 w1160] -> w1124
                  tunnel: [w1134 w1159] -> w1123
                  tunnel: w1121 -> [w1135 _]
                  tunnel: w1122 -> [w1136 w1158]
                  tunnel: [w1131 w1158] -> w1120
                  tunnel: [w1130 TRUE] -> w1119
                  tunnel: w1116 -> [w1128 _]
                  frame False {
                    # "Backward (F-E)"
                    n549 = Less Or Equal?(x=w1129, y=w1128) -> (x <= y?=w1137:bool)
                    n550 = case shown="True" w1137 {
                      tunnel: w1136 -> [w1140 w1150]
                      tunnel: w1135 -> [_ w1149]
                      tunnel: [FALSE w1147] -> w1134
                      tunnel: w1133 -> [w1142 w1145]
                      tunnel: [w1141 w1146] -> w1132
                      tunnel: [w1140 w1144] -> w1131
                      tunnel: [TRUE w1143] -> w1130
                      frame False {
                        # "Hasn't reached\n-continue"
                        n551 = Negate(x=w1142) -> (-x=w1141:dbl)
                      }
                      frame True {
                        # "Back at start"
                        n552 = Increment(x=w1150) -> (x+1=w1144:i32)
                        n553 = Greater Or Equal?(x=w1144, y=w1149) -> (x >= y?=w1148:bool)
                        n554 = case shown="False" w1148 {
                          tunnel: [TRUE TRUE] -> w1147
                          tunnel: [w1152 0.0] -> w1146
                          tunnel: w1145 -> [w1152 _]
                          tunnel: [TRUE FALSE] -> w1143
                          frame False {
                            # "Next sweep"
                          }
                          frame True {
                            # "Sweeps Complete"
                          }
                        }
                      }
                    }
                  }
                  frame True {
                    # "Forward (E-F)"
                    n555 = Greater Or Equal?(x=w1164, y=w1163) -> (x >= y?=w1162:bool)
                    n556 = case shown="False" w1162 {
                      tunnel: w1161 -> [w1166 w1169]
                      tunnel: [w1166 w1168] -> w1160
                      tunnel: [TRUE FALSE] -> w1159
                      frame False {
                        # "Hasn't reached\n-continue"
                      }
                      frame True {
                        # "Hit full\n-turn-around"
                        n557 = Negate(x=w1169) -> (-x=w1168:dbl)
                      }
                    }
                  }
                }
              }
              frame Enabled {
                n558 = Increment(x=w1182) -> (x+1=w1180:i32)
                n559 = Greater Or Equal?(x=w1180, y=w1181) -> (x >= y?=w1175:bool)
                n560 = case shown="True" w1175 {
                  tunnel: w1174 -> [w1184 w1188]
                  tunnel: w1173 -> [_ w1186]
                  tunnel: [w1184 w1187] -> w1172
                  tunnel: [TRUE w1185] -> w1171
                  frame False {
                    # "Same Sweep"
                  }
                  frame True {
                    # "Sweep Ended"
                    n561 = Increment(x=w1188) -> (x+1=w1187:i32)
                    n562 = Less?(x=w1187, y=w1186) -> (x < y?=w1185:bool)
                  }
                }
                n563 = Select(t=0, s=w1175, f=w1180) -> (s? t:f=w1170:i32)
                n564 = Index Array(array=w1177, index=w1170) -> (element=w1176:dbl)
              }
            }
            n565 = Insert Into Array(array=w1104, index=0, new element=string[] ["Write Controls"]) -> (w1103:string[])
            n566 = Replace Array Subset(array=w1114, new element=w1111, index=0) -> (w1098:dbl[])
            n567 = Index Array(array=w1098) -> (element #1=w1101:dbl, element #2=w1100:dbl, element #3=w1099:dbl)  [unwired: 3 in]
            n568 = Bundle By Name(cluster=w1110, "Controls"=w1098, "SweepsForward"=w1108, "SweepsSwept"=w1105, "Current Point"=w1088, "SweepsRunning"=w1096) -> (w1109:T12)
            n569 = local write "pb.RunSweeps"(w1096) -> ()
            n570 = local write "Spare Output"(w1099) -> ()
            n571 = local write "Cal Controls:"(w1098) -> ()
            n572 = local write "PS Command"(w1100) -> ()
            n573 = local write "Position Command"(w1101) -> ()
          }
          frame Enabled {
          }
        }
      }
      frame "Save Sweeps" {
        n574 = Unbundle By Name(w1204) -> ("Graph Data"=w1191:dbl[][], "New Data"=w1196:bool, "Data Path"=w1201:path, "Data"=w1200:dbl[][], "Data Index"=w1202:i32, "Test Params.Bias Resistance"=w1199:dbl, "MaxResistance"=w1194:dbl, "FinalizeSweeps"=w1195:bool, "Max Height"=w1193:dbl, "Min Height"=w1192:dbl)
        n575 = case shown="True" w1196 {
          tunnel: w1204 -> [w1214 w1258]
          tunnel: [w1214 w1257] -> w1203
          tunnel: w1202 -> [_ w1251]
          tunnel: w1201 -> [_ w1245]
          tunnel: w1200 -> [_ w1244]
          tunnel: w1199 -> [_ w1242]
          tunnel: w1194 -> [_ w1229]
          tunnel: w1193 -> [_ w1221]
          tunnel: w1192 -> [_ w1222]
          tunnel: w1191 -> [_ w1217]
          frame False {
          }
          frame True {
            # "Changed from 0.0005"
            # "Time Elapsed\nLS Voltage\nPS Voltage\nHeight\nLS Resistance"
            # "PS Voltage\nLS Voltage\nSpare\nAbs. Height\nRel. Height"
            n576 = Index Array(array=w1244, index (col) #1=4 ("disabled index (col)"), index (col) #2=1 ("index (col)"), index (col) #3=0 ("index (col)")) -> (element #1=w1227:dbl[], element #2=w1231:dbl[], element #3=w1230:dbl[])  [unwired: 3 in]
            n577 = for {
              tunnel: w1231 -> [w1269] mode=indexing
              tunnel: w1230 -> [w1273] mode=indexing
              tunnel: w1242 -> [w1268]
              tunnel: [w1266] -> w1241 mode=indexing
              shift-right: [w1264] -> w1228
              shift-left: w1229 -> [w1265]
              n578 = Subtract(x=w1273, y=w1269) -> (x-y=w1270:dbl)
              n579 = Equal To 0?(x=w1270) -> (x = 0?=w1272:bool)
              n580 = Not A Number/Path/Refnum?(number/path/refnum=w1268) -> (NaN/Path/Refnum?=w1271:bool)
              n581 = Or(x=w1272, y=w1271) -> (x .or. y?=w1267:bool)
              n582 = case shown="False" w1267 {
                tunnel: w1270 -> [_ w1285]
                tunnel: w1269 -> [_ w1284]
                tunnel: w1268 -> [_ w1282]
                tunnel: ["NaN" w1280] -> w1266
                tunnel: w1265 -> [w1274 w1277]
                tunnel: [w1274 w1279] -> w1264
                frame True {
                }
                frame False {
                  n583 = Divide(x=w1284, y=w1285) -> (x/y=w1283:dbl)
                  n584 = Multiply(x=w1283, y=w1282) -> (x*y=w1278:dbl)
                  n585 = Greater?(x=w1277, y=w1278) -> (0:w1276:bool)
                  n586 = Select(t=w1277, s=w1276, f=w1278) -> (s? t:f=w1279:dbl)
                  n587 = Number To Fractional String(number=w1278, precision (6)=i16 3) -> (F-format string=w1280:string)  [unwired: 2 in]
                }
              }
            }
            n588 = Array Size(array=w1230) -> (size(s)=w1256:i32)
            n589 = Add(x=w1256, y=w1251) -> (x+y=w1255:i32)
            n590 = for {
              N: w1256 -> [_]
              tunnel: w1251 -> [w1292]
              tunnel: [w1286] -> w1247 mode=indexing
              i -> [w1291]
              n591 = Add(x=w1292, y=w1291) -> (x+y=w1289:i32)
              n592 = Multiply(x=w1289, y=0.001) -> (x*y=w1288:dbl)
              n593 = Number To Fractional String(number=w1288, precision (6)=i16 4) -> (F-format string=w1286:string)  [unwired: 2 in]
            }
            n594 = Number To Fractional String(number=w1230, precision (6)=i16 3) -> (F-format string=w1248:string[])  [unwired: 2 in]
            n595 = Number To Fractional String(number=w1231, precision (6)=i16 3) -> (F-format string=w1249:string[])  [unwired: 2 in]
            n596 = Number To Fractional String(number=w1227, precision (6)=i16 3) -> (F-format string=w1250:string[])  [unwired: 2 in]
            n597 = Build Array(w1247, w1250, w1249, w1248, w1241) -> (w1243:string[][])
            n598 = Array Max & Min(array=w1227) -> (max value=w1225:dbl, min value=w1223:dbl)  [unwired: 2 out]
            n599 = Transpose 2D Array(2D array=w1243) -> (transposed array=w1218:string[][])
            n600 = Open/Create/Replace File(file path (use dialog)=w1245, operation (0:open)=T19."open") -> (refnum out=w1236:refnum<file>, error out=w1235:errorcluster)  [unwired: 4 in, 1 out]
            n601 = Greater?(x=w1225, y=w1221) -> (0:w1226:bool)
            n602 = Less?(x=w1223, y=w1222) -> (x < y?=w1224:bool)
            n603 = Fract/Exp String To Number(string=w1218) -> (number=w1216:dbl[][])  [unwired: 3 in, 1 out]
            n604 = Set File Position(refnum=w1236, from (0:start)=enum16{"start", "end", "current"}."end", error in=w1235) -> (refnum out=w1233:refnum<file>, error out=w1232:errorcluster)  [unwired: 1 in]
            n605 = Array To Spreadsheet String(delimiter (Tab)=",", array=w1218, 3:"%s" ("format string")) -> (spreadsheet string=w1246:string)
            n606 = Build Array (concatenate)(w1217, w1216) -> (w1215:dbl[][])
            n607 = Select(t=w1225, s=w1226, f=w1221) -> (s? t:f=w1219:dbl)
            "Max Height" <- w1219
            n608 = Select(t=w1223, s=w1224, f=w1222) -> (s? t:f=w1220:dbl)
            "Min Height" <- w1220
            n609 = Write to Text File(file (use dialog)=w1233, text=w1246, error in=w1232) -> (refnum out=w1239:refnum<file>, error out=w1240:errorcluster)  [unwired: 1 in, 1 out]
            n610 = Close File(refnum=w1239, error in=w1240) -> (error out=w1238:errorcluster)  [unwired: 1 out]
            n611 = Bundle By Name(cluster=w1258, "Graph Data"=w1215, "Data Index"=w1255, "MaxResistance"=w1228, "Max Height"=w1219, "Min Height"=w1220) -> (w1257:T12)
            n612 = call <vilib>:"Clear Errors.vi"("error in (no error)"=w1238) -> ()  [unwired: 5 in, 2 out]
          }
        }
        n613 = disable-structure shown="Enabled" {
          disable-tunnel: w1198 -> [w1207 w1213]
          disable-tunnel: [w1206 w1213] -> w1197
          disable-tunnel: w1195 -> [w1205 _]
          frame Disabled {
            n614 = case shown="True" w1205 {
              tunnel: w1207 -> [w1208 w1212]
              tunnel: [w1208 w1211] -> w1206
              frame False {
              }
              frame True {
                n615 = Insert Into Array(array=w1212, index=0, new element="Finalize Sweeps" ("new element/subarray")) -> (w1211:string[])
              }
            }
          }
          frame Enabled {
          }
        }
      }
      frame "Finalize Sweeps" {
        w1295 = FALSE ("Graph Active")
        # "Handle shutting off PS before transferring file to specified (generally network) location"
        # "Done because network lag was causing issues"
        # "Split into 2 parts now that using a temporary file, and tranferring after finished, but before handing to graph script"
        n616 = Unbundle By Name(w1297) -> ("Controls"=w1296:dbl[])
        n617 = Replace Array Subset(array=w1296, new element=0.0 ("new element/subarray"), index=1) -> (w1303:dbl[])
        n618 = Index Array(array=w1303) -> (element #1=w1302:dbl, element #2=w1301:dbl, element #3=w1300:dbl)  [unwired: 3 in]
        n619 = Insert Into Array(array=w1306, index=0, new element=string[] ["Write Controls", "Finalize Sweeps 2"]) -> (w1305:string[])
        n620 = property on="pb.RunSweeps" class="Bool (strict)"("DisabledEnum"=T20."Disabled and Grayed Out" ("Disabled")) -> ()  [unwired: 2 in, 2 out]
        n621 = Bundle By Name(cluster=w1297, "Graph Active"=w1295, "Controls"=w1303) -> (w1294:T12)
        n622 = local write "Spare Output"(w1300) -> ()
        n623 = local write "Cal Controls:"(w1303) -> ()
        n624 = local write "PS Command"(w1301) -> ()
        n625 = local write "Position Command"(w1302) -> ()
        n626 = local write "pb.graph control"(w1295) -> ()
      }
      frame "Finalize Sweeps 2" {
        # "Done because network lag was causing issues"
        # "Split into 2 parts now that using a temporary file, and tranferring after finished, but before handing to graph script"
        n627 = Unbundle By Name(w1323) -> ("Graph Data"=w1308:dbl[][], "Data Path"=w1309:path, "Test Params.Test Header.CA Number:"=w1321:string, "Test Params.Test Header.Part Model:"=w1320:string, "Test Params.Test Header.Hours Description:"=w1319:string, "Test Params.Test Header.Part Serial Number:"=w1316:string, "Test Params.Test Style"=w1314:T2, "Test Params.Graph Parameters"=w1311:T3)
        n628 = property on="pb.Re-Run Graph" class="Bool"("DisabledEnum"=T20."Enabled" ("Disabled")) -> ()  [unwired: 2 in, 2 out]
        n629 = Format Into String(w1314) -> (resulting string=w1313:string)  [unwired: 3 in, 1 out]
        n630 = Format Into String(format string="%s, %s, %s", w1321, w1320, w1319) -> (resulting string=w1317:string)  [unwired: 2 in, 1 out]
        n631 = Format Into String(format string="%s, %s", w1316, w1313) -> (resulting string=w1312:string)  [unwired: 2 in, 1 out]
        n632 = call "Graphing Data (global).vi"("Data"=w1308, "Data Path"=w1309, "Title 1"=w1317, "Title 2"=w1312, "Graph Parameters"=w1311, "Mode"=enum16{"Read", "Write", "Init", "Stop"}."Write") -> ()  [unwired: 7 in, 7 out]
        n633 = Insert Into Array(array=w1327, index=0, new element=string[] ["Handle Enables"]) -> (w1326:string[])
      }
      frame "Freeze Screen" {
        n634 = control-ref of="This VI"() -> (w1330:refnum<vi>)
        n635 = property class="VI"(reference=w1330) -> ("Panel"=w1329:refnum<vi>)  [unwired: 1 in, 2 out]
        n636 = property class="Pnl"(reference=w1329, "DeferPanUpdts"=TRUE ("Defer Panel Updates")) -> ()  [unwired: 1 in, 2 out]
      }
      frame "Thaw Screen" {
        n637 = control-ref of="This VI"() -> (w1337:refnum<vi>)
        n638 = property class="VI"(reference=w1337) -> ("Panel"=w1336:refnum<vi>)  [unwired: 1 in, 2 out]
        n639 = property class="Pnl"(reference=w1336, "DeferPanUpdts"=FALSE ("Defer Panel Updates")) -> ()  [unwired: 1 in, 2 out]
      }
      frame "Save Config" {
        n640 = Unbundle By Name(w1343) -> ("Config Path"=w1342:path, "Config"=w1340:T10)
        n641 = call <vilib>:"Open Config Data.vi"("configuration file path"=w1342) -> ("refnum"=w1341:T25)  [unwired: 8 in, 2 out]
        n642 = call <userlib>:"Write INI Cluster__ogtk.vi"("INI Fomatted Cluster"=w1340, "refnum"=w1341) -> ("error out"=w1338:errorcluster, "dup refnum"=w1339:T25)  [unwired: 8 in]
        n643 = call <vilib>:"Close Config Data.vi"("error in (no error)"=w1338, "refnum"=w1339) -> ()  [unwired: 8 in, 2 out]
      }
      frame "RIO Connection" {
        n644 = disable-structure shown="Disabled" {
          disable-tunnel: w1348 -> [w1352 w1403]
          disable-tunnel: [w1351 w1403] -> w1347
          disable-tunnel: w1346 -> [w1350 w1404]
          disable-tunnel: [w1349 w1404] -> w1345
          frame Disabled {
            n645 = while {
              tunnel: w1352 -> [w1356]
              tunnel: [w1355] -> w1351
              shift-right: [w1353] -> w1349
              shift-left: w1350 -> [w1354]
              stop <- w1357 stop-if-true
              n646 = event shown="[2]" {
                selector: _ -> [_ _ _ _]
                dyn-events: _ -> [_ _ _ _]
                timeout: 50 -> [_ _ _ _]
                tunnel: [FALSE TRUE ("Discard?") TRUE TRUE ("Discard?")] -> w1357
                tunnel: [w1360 w1363 w1392 string[] ["Exit Preparation"]] -> w1353
                tunnel: w1356 -> [w1361 w1368 w1396 w1400]
                tunnel: [w1361 w1367 w1396 w1400] -> w1355
                tunnel: w1354 -> [w1360 w1366 w1395 _]
                event Timeout {
                  n647 = event-data() -> ()  [unwired: 1 in, 1 out]
                  n648 = local write "Screen"(T21."RIO Connection" ("Screen")) -> ()
                }
                event #1 (no event record) {
                  n649 = event-data() -> ("NewVal"=w1369)  [unwired: 1 in]
                  n650 = String Length(string=w1369) -> (length=w1379:i32)
                  n651 = Search and Replace String(replace all?=TRUE ("replace all? (F)"), input string=w1369, search string=".") -> (number of replacements=w1373:i32)  [unwired: 5 in, 3 out]
                  n652 = In Range and Coerce(upper limit=15, x=w1379, lower limit=7) -> (In Range?=w1374:bool)  [unwired: 1 out]
                  n653 = Equal?(x=w1373, y=3) -> (x = y?=w1371:bool)
                  n654 = And(x=w1371, y=w1374) -> (x .and. y?=w1370:bool)
                  n655 = case shown="True" w1370 {
                    tunnel: w1369 -> [_ w1383]
                    frame False {
                    }
                    frame True {
                      n656 = Current VI's Path() -> (path=w1387:path)
                      n657 = Strip Path(path=w1387) -> (stripped path=w1386:path)  [unwired: 1 out]
                      n658 = Build Path(base path=w1386, name or relative path="IP.ini") -> (appended path=w1384:path)
                      n659 = call <vilib>:"Open Config Data.vi"("configuration file path"=w1384) -> ("error out"=w1390:errorcluster, "refnum"=w1388:T25)  [unwired: 8 in, 1 out]
                      n660 = call-poly <vilib>:"Write Key.vi"("section"="IP", "error in (no error)"=w1390, "value"=w1383, "key"="IP Address", "refnum"=w1388) -> ("error out"=w1381:errorcluster, "refnum out"=w1382:T25)  [unwired: 4 in, 1 out]
                      n661 = local write "IP Address"(w1383) -> ()
                      n662 = call <vilib>:"Close Config Data.vi"("error in (no error)"=w1381, "refnum"=w1382) -> ()  [unwired: 8 in, 2 out]
                    }
                  }
                  n663 = Bundle By Name(cluster=w1368, "IP Address"=w1369) -> (w1367:T12)
                  n664 = Insert Into Array(array=w1366, index=0, new element=string[] ["Save Config", "RIO Connection"]) -> (w1363:string[])
                }
                event #2 (no event record) {
                  w1397 = "Connecting" ("Boolean Text.Text")
                  n665 = event-data() -> ()  [unwired: 1 in, 1 out]
                  n666 = local read item#-1() -> (w1398)
                  n667 = local write "IP Address"(w1398) -> ()
                  n668 = Insert Into Array(array=w1395, index=0, new element=string[] ["Set Cursor Busy", "Request Connection", "Connect to RIO"]) -> (w1392:string[])
                }
                event "Panel Close?": Value Change {
                  n669 = event-data() -> ()  [unwired: 1 in, 1 out]
                }
              }
            }
          }
          frame Enabled {
          }
        }
      }
      frame "Request Connection" {
        w1417 = T26 {"ConnectAttemptLimit(5)"=5, "IP Address"="", "Send Port"=0, "Recv Port"=0}  # ConnSettingCluster
        # "The calibration software creates ports based on last section of RIO IP address plus 5000\nsince our section start at 100 these ports are fine for now... should possibly do the same thing with a different base"
        n670 = Unbundle By Name(w1406) -> ("Config.RT IP Address"=w1405:string)
        "IP Address" <- w1405
        n671 = Bundle(cluster=w1417, "ConnectAttemptLimit(5)"=u32 5, "IP Address"=w1405, "Send Port"=u16 5555, "Recv Port"=u16 5050) -> (w1416:T26)
        n672 = Flatten To String(anything=w1416) -> (data string=w1415:string, error out=w1408:errorcluster)  [unwired: 3 in, 1 out]
        n673 = call "PC Send Event.vi"("PC Send Command"=PCsend_RTrecv_CMD."ConnSettings", "Mode"=Event_Mode."Set", "Flattened Data"=w1415, "Error In"=w1408) -> ("Error Out"=w1409:errorcluster)  [unwired: 10 in, 1 out]
        n674 = call "PC Send Event.vi"("PC Send Command"=PCsend_RTrecv_CMD."Connect", "Mode"=Event_Mode."Set", "Error In"=w1409) -> ("Error Out"=w1407:errorcluster)  [unwired: 11 in, 1 out]
        n675 = call <vilib>:"Clear Errors.vi"("error in (no error)"=w1407) -> ()  [unwired: 5 in, 2 out]
      }
      frame "Handle Disables", "Handle Enables" {
        n676 = case shown="\"Handle Disables\"" w1422 {
          tunnel: [T20."Enabled" ("Disabled") T20."Disabled and Grayed Out" ("Disabled")] -> w1421
          frame "Handle Enables", Default {
          }
          frame "Handle Disables" {
          }
        }
        n677 = property on="Sweep Start Height" class="DigNum (strict)"("DisabledEnum"=w1421) -> ()  [unwired: 2 in, 2 out]
        n678 = property on="Sweep End Height" class="DigNum (strict)"("DisabledEnum"=w1421) -> ()  [unwired: 2 in, 2 out]
        n679 = property on="Sweep Time (s)" class="DigNum (strict)"("DisabledEnum"=w1421) -> ()  [unwired: 2 in, 2 out]
        n680 = property on="Sweep PS Cmd" class="DigNum (strict)"("DisabledEnum"=w1421) -> ()  [unwired: 2 in, 2 out]
        n681 = property on="Number of Sweeps" class="DigNum (strict)"("DisabledEnum"=w1421) -> ()  [unwired: 2 in, 2 out]
        n682 = property on="Position Command" class="DigNum (strict)"("DisabledEnum"=w1421) -> ()  [unwired: 2 in, 2 out]
        n683 = property on="PS Command" class="DigNum (strict)"("DisabledEnum"=w1421) -> ()  [unwired: 2 in, 2 out]
        n684 = property on="Spare Output" class="DigNum (strict)"("DisabledEnum"=w1421) -> ()  [unwired: 2 in, 2 out]
        n685 = property on="pb.CalPage" class="Bool"("DisabledEnum"=w1421) -> ()  [unwired: 2 in, 2 out]
        n686 = property on="pb.TareHeight" class="Bool"("DisabledEnum"=w1421) -> ()  [unwired: 2 in, 2 out]
        n687 = property on="Test Header Tab" class="TabCtl (strict)"("DisabledEnum"=w1421) -> ()  [unwired: 2 in, 2 out]
        n688 = property on="Test Setup Tab" class="TabCtl (strict)"("DisabledEnum"=w1421) -> ()  [unwired: 2 in, 2 out]
        n689 = property on="Graph Setup Tab" class="TabCtl (strict)"("DisabledEnum"=w1421) -> ()  [unwired: 2 in, 2 out]
      }
      frame "Set Cursor Busy" {
        n690 = call <vilib>:"Set Busy.vi"() -> ()  [unwired: 10 in, 2 out]
      }
      frame "Unset Cursor Busy" {
        n691 = call <vilib>:"Unset Busy.vi"() -> ()  [unwired: 11 in, 1 out]
      }
      frame "EXIT" {
        n692 = property class="App"() -> ("App.Kind"=w1434:T16)  [unwired: 2 in, 2 out]
        n693 = case shown="Default" w1434 {
          frame Default {
            n694 = control-ref of="This VI"() -> (w1438:refnum<vi>)
            n695 = invoke class="VI" method="FP.Close"(reference=w1438) -> ()  [unwired: 2 in, 3 out]
          }
          frame "Development System" {
          }
        }
        n696 = call "PC Send Event.vi"("PC Send Command"=PCsend_RTrecv_CMD."Stop", "Mode"=Event_Mode."Set") -> ()  [unwired: 12 in, 2 out]
        n697 = call "Graphing Data (global).vi"("Mode"=enum16{"Read", "Write", "Init", "Stop"}."Stop") -> ()  [unwired: 12 in, 7 out]
      }
    }
  }
  n698 = call "PC Engine.vi"("Error In"=w11) -> ("Error Out"=→"Error Out":errorcluster, "InvalidResponses"=→"InvalidResponses":string)  [unwired: 3 in]
  n699 = flat-sequence {
    tunnel: w11 -> [w1440]
    tunnel: [w1440] -> w10
    tunnel: w9 -> [w1439]
    tunnel: w10 -> [w1442]
    frame #0 {
      n700 = Wait on Occurrence(2:w1439) -> ()  [unwired: 2 in, 1 out]
    }
    frame #1 {
      n701 = while {
        shift-right: [w1449] -> _
        shift-left: _ -> [w1448]
        shift-right: [w1443] -> _
        shift-left: string[] ["Connect"] -> [w1452]
        tunnel: w1442 -> [_]
        stop <- w1446 stop-if-true
        n702 = local read "Panel Close?"() -> (w1446:bool)
        n703 = Delete From Array(array=w1452, index=0) -> (deleted portion=w1447:string, array with subset deleted=w1451:string[])  [unwired: 1 in]
        n704 = Select(t="Stop" ("string"), s=w1446, f=w1447) -> (s? t:f=w1444:string)
        n705 = case shown="\"Connect\", Default" w1444 {
          tunnel: w1451 -> [w1458 w1490 w1501]
          tunnel: [w1453 w1484 refnum<k21> refnum ("reader name")] -> w1449
          tunnel: w1448 -> [_ w1483 w1502]
          tunnel: [w1457 w1489 w1501] -> w1443
          frame "Connect", Default {
            n706 = local read "IP Address"() -> (w1456:string)
            n707 = Concatenate Strings("//" ("string"), w1456, "/writer" ("string")) -> (w1463:string)
            n708 = Create Network Stream Reader Endpoint(5:250 ("timeout in ms (-1)"), 7:4096 ("timeout in ms (-1)"), 9:0.0, 10:w1463, 11:"reader" ("reader name")) -> (0:w1460:errorcluster, 3:w1454:refnum<k21>)  [unwired: 2 in]
            n709 = Unbundle By Name(w1460) -> ("status"=w1459:bool)
            n710 = case shown="False" w1459 {
              tunnel: w1458 -> [w1469 w1477]
              tunnel: [w1468 w1476] -> w1457
              tunnel: w1454 -> [w1467 w1472]
              tunnel: [w1467 w1472] -> w1453
              frame False {
                # "Connected"
                n711 = Insert Into Array(array=w1469, index=0, new element=string[] ["Data"]) -> (w1468:string[])
              }
              frame True {
                # "Error"
                n712 = Insert Into Array(array=w1477, index=0, new element=string[] ["Connect"]) -> (w1476:string[])
                n713 = Wait (ms)(milliseconds to wait=u32 100) -> ()  [unwired: 1 out]
              }
            }
          }
          frame "Data" {
            n714 = property class="Network Stream Endpoint"(reference=w1483) -> (reference out=w1481:refnum<k21>, error out=w1480:errorcluster, "AvailElmntsForRead"=w1479:i32)  [unwired: 1 in]
            n715 = case shown="Default" w1479 {
              tunnel: [w1493 w1496] -> w1491
              tunnel: [w1494 w1499] -> w1484
              tunnel: w1481 -> [w1494 w1498]
              tunnel: w1480 -> [w1493 w1497]
              frame 0 {
                n716 = call "Data (Global).vi"("Mode"=T17."Write Stream Error", "Write Stream Error"=w1493) -> ()  [unwired: 10 in, 4 out]
              }
              frame Default {
                n717 = shared-variable-read(w1498, w1497) -> (w1499:refnum<k21>, w1496:errorcluster, w1500:dbl[])  [unwired: 2 in, 1 out]
                n718 = call "Data (Global).vi"("Data In"=w1500, "Mode"=T17."Write Data", "Write Stream Error"=w1496) -> ()  [unwired: 9 in, 4 out]
              }
            }
            n719 = Unbundle By Name(w1491) -> ("status"=w1478:bool)
            n720 = Wait (ms)(milliseconds to wait=u32 50) -> ()  [unwired: 1 out]
            n721 = Select(t="Connect", s=w1478, f="Data") -> (s? t:f=w1485:string)
            n722 = Insert Into Array(array=w1490, index=0, new element=w1485) -> (w1489:string[])
          }
          frame "Stop" {
            n723 = Destroy Stream Endpoint(11:w1502) -> ()  [unwired: 1 in, 1 out]
          }
        }
      }
    }
  }
  n724 = while {
    tunnel: w11 -> [_]
    stop <- w1504 stop-if-true
    n725 = event shown="[0] Timeout" {
      selector: _ -> [_ _]
      dyn-events: _ -> [_ _]
      timeout: 100 -> [_ _]
      tunnel: [FALSE w1507] -> w1504
      event Timeout {
        n726 = event-data() -> ()  [unwired: 1 in, 1 out]
      }
      event Panel Close? {
        w1507 = TRUE ("Discard?")
        n727 = event-data() -> ()  [unwired: 1 in, 1 out]
        n728 = property on="Panel Close?" class="Bool (strict)"("Val(Sgnl)"=w1507) -> ()  [unwired: 2 in, 2 out]
        n729 = event-data("Discard?"=w1507) -> ()  [unwired: 1 in, 1 out]
      }
    }
  }
